vi "main 1.12 stable LR.vi"() -> ()   [LabVIEW 2020]
uses:
  subvi/Newport ESP301/Newport ESP301.lvlib
  subvi/sp_manip.llb/sp_manip_lib.lvlib
  subvi/sp_manip.llb/tcp_gateway.lvlib
  subvi/PHOIBOS/DEFINITIONS/DEF_dev_type.ctl
  subvi/PHOIBOS/DEFINITIONS/DEF_dev_state.ctl
  <vilib>/Utility/file.llb/Write Delimited Spreadsheet (DBL).vi
  <vilib>/Analysis/NI_AALBase.lvlib
  <vilib>/Analysis/1siggen.llb/Ramp Pattern by Samples.vi
  <vilib>/Analysis/NI_AALPro.lvlib
  <vilib>/Analysis/_algsub.llb/Real Vector Norm.vi
  subvi/ZaberTSeries/ZaberTSeries.lvlib
  <vilib>/Utility/file.llb/Write Delimited Spreadsheet (string).vi
  <vilib>/DAQmx/create/channels.llb/DAQmx Create Channel (DI-Digital Input).vi
  <vilib>/Utility/file.llb/Read Delimited Spreadsheet (string).vi
panel:
  out "Pics L":i32=20
  out "Waveform Chart":dbl(graph)
  out "G2 X":cluster{dbl[], "Ramp Pattern":dbl[]}(graph)
  in  "reset every n pics":bool=TRUE
  in  "pics2avg":i32=50
  in  "abort acq.":bool
  out "G2 Y":cluster{dbl[], "Ramp Pattern":dbl[]}(graph)
  out "ETA":timestamp=timestamp(3553173084.423481 s since 1904-01-01) format="%<%H:%M:%S>T"
  out "acq. imgs":i32=20
  out "snap_prog":dbl(slide)=1.0 scale=0.0..1.0
  in  "BasePath":path=path "Z:/PESdata"
  in  "cam_liveavg":bool=TRUE caption="live average"
  out "cam_fps":dbl=19.778711584654577 caption="FPS" format="%.1g"
  out "sideimg":dbl[][](graph)
  out "RunNumber":u16=1876
  out "sum":dbl format="%#.2g"
  out "max":dbl
  out "mainimg":dbl[][](graph)
  out "ESP_con?":bool=TRUE caption="ESP301"
  out "phoib_con?":bool caption="PHOIBOS"
  out "manip_con?":bool=TRUE caption="manipulator"
  out "cam_con?":bool caption="camera"
  in  "main_close":bool
  in  "Tab Control":enum32{"live", "1D scan", "devices"}(tab)=enum."devices"
  in  "phoib_I_10s":dbl=0.0039
  out "phoib_I_10":dbl caption="Mesh Back"
  in  "mirr_go":bool
  in  "ESP_opent0file":bool
  in  "mirr_rel":i32=20 caption="relative [steps]"
  in  "mirr_Y-":bool
  in  "mirr_Y+":bool
  in  "mirr_X+":bool
  in  "mirr_X-":bool
  in  "manip_deltas":dbl[](array[numeric])=[0.0, 0.0, 5.0, 0.0, 0.0, 0.0] caption="delta" format="%#.5g"
  in  "aq.mode":enum32{"Radio Selection 1", "Radio Selection 2"}(radio)=enum."Radio Selection 2"
  in  "dark avg":i32=100
  in  "cam_avgs":i32=20 caption="N"
  in  "ESP_delta":dbl caption="relative [mm]"
  in  "ESP_-":bool
  in  "ESP_+":bool
  in  "ESP_go":bool
  in  "ESP_dest_t":dbl=-12656.75602819869 caption="[fs]"
  in  "ESP_dest":dbl=25.0 caption="[mm]"
  in  "ESP_set_t0":bool
  in  "phoib_I_6s":dbl=3200.0
  in  "phoib_I_5s":dbl=1500.0
  in  "phoib_I_4s":dbl=4.558
  in  "phoib_I_3s":dbl=-7.0
  in  "phoib_I_2s":dbl=30.0
  in  "phoib_I_1s":dbl=18.0
  in  "phoib_standby":bool
  in  "phoib_set":bool
  out "phoib_I_6":dbl caption="Screen Voltage"
  out "phoib_I_5":dbl caption="Detctor Voltage"
  out "phoib_I_4":dbl caption="Work Function"
  out "phoib_I_3":dbl caption="Coil Current"
  out "phoib_I_2":dbl caption="Pass Energy"
  out "phoib_I_1":dbl caption="Kinetic Energy"
  out "Saved Positions":string[][](table)=[["ertwertwert", "-2.299945", "-2.030214", "38.900024", "50.000762", "0.000887", "-97.998082"], ["uztgugt", "-14.999451", "-13.638894", "442.380066", "13.998380", "-1.893758", "-76.305838"], ["asdf", "-14.999451", "-13.638894", "442.380066", "13.998380", "-1.893758", "-76.305838"], ["test3", "-14.999451", "-13.638894", "441.380066", "13.998380", "-1.893758", "-76.305838"]]
  in  "Save Pos":bool
  in  "Load":bool
  in  "Delete":bool
  in  "ManipRel +":bool
  in  "ManipRel -":bool
  in  "Move Abs":bool
  in  "stop manip":bool
  in  "dest":dbl[](array[numeric])=[-0.09886108403264701, -4.840202394941505, 34.40008544921875, 285.0011913575033, -7.998926328051604, 138.99937717186526] caption="destination" format="%#.5g"
  out "axis":string[](array[string])=["x", "y", "z", "polar", "tilt", "azimut"]
  out "pos":dbl[](array[numeric])=[-0.09886108403264701, -4.840202394941505, 34.40008544921875, 285.0011913575033, -7.998926328051604, 138.99937717186526] caption="position" format="%.5f"
  in  "ana_mode":T1(ring)=enum."WideAngleMode"
  in  "ana_voltrange":enum16{"3.5kV", "1.5kV", "400V", "100V", "10V"}(ring)=enum."400V"
  out "ESP_pos":dbl=nan caption="Position"
  out "ESP_delay":dbl=nan caption="Delay"
  out "ESP_t0":dbl=25.0 caption="Time Zero @"
  out "phoib_I_7":dbl caption="Conversion Voltage"
  in  "phoib_I_7s":dbl=-26.0
  in  "phoib_I_8s":dbl=0.0039
  in  "phoib_I_9s":dbl=0.0039
  out "phoib_I_8":dbl caption="FD1"
  out "phoib_I_9":dbl caption="Mesh Front"
  in  "gain":bool
  in  "cam_exp":u32=50 caption="exposure [ms]"
  in  "binning":u16(ring)=2 items=["X 1", "X 2", "X 4", "X 8"]
  in  "cam_dark?":bool=TRUE caption="subtract dark?"
  in  "cam_dark":bool
  in  "cam_saveimg":bool
  in  "e-size":u8
  in  "lower threshold":i32=50
  in  "count?":bool
  in  "ROI Left":i32=1
  in  "ROI Right":i32=43
  in  "ROI Top":i32=1
  in  "ROI Bottom":i32=33
  out "moving?":bool[](array[boolean])
  out "mirr_posX":i32=-142 caption="X"
  out "mirr_posY":i32=4922 caption="Y"
  in  "mirr_dest":i32[](array[numeric])=[-64, -2601]
  out "anglegraph":dbl[][](graph)
  out "intensitygraph":cluster{"Array":dbl[], "Intensity Chart":dbl[]}(graph)={"Array"=[-100000.0, -95000.0, -90000.0, -85000.0, -80000.0, -75000.0, -70000.0, -65000.0, -60000.0, -55000.0, -50000.0, -45000.0, -40000.0, -35000.0, -30000.0, -25000.0, -20000.0, -15000.0, -10000.0, -5000.0, 0.0, 5000.0, 10000.0, 15000.0, 20000.0, 25000.0, 30000.0, 35000.0, 40000.0, 45000.0, 50000.0], "Intensity Chart"=[710968.0999999978, 661453.8299999974, 660491.1499999983, 654490.9100000008, 607000.039999999, 668861.0999999981, 631366.7699999984, 739689.6549999982, 681310.9099999986, 658872.4599999987, 692812.8950000014, 671304.7250000003, 670701.9799999978, 684100.4049999971, 706126.3150000001, 744782.0600000009, 684440.8499999981, 704157.155, 756957.4599999988, 768506.4449999956, 761428.5800000022, 678039.9949999974, 735774.9649999988, 659533.465000001, 724648.9199999974, 705546.0750000002, 773026.2399999972, 698578.0149999986, 697856.3899999985, 787613.0450000013, 750231.4800000007]}
  in  "scan_selector":enum32{"delay", "manip", "mirror", "volt"}(tab)
  in  "scan_manip_setstart":bool
  in  "scan_manip_start":dbl[](array[numeric])=[-2.6172862113166087, -0.009888298846365134, 68.5008544921875, -46.363686276590336, 11.108982061941884, -218.56360350415366] caption="start position" format="%#.5g"
  in  "scan_manip_deltas":dbl[](array[numeric])=[0.0, 0.0, 0.0, 0.0, 10.0, 0.0] caption="direction vector\n(gets normed)" format="%#.5g"
  in  "scan_mirr_start":i32[](array[numeric])=[-64, -2601]
  in  "scan_mirr_deltas":i32[](array[numeric])=[0, 0, 0, 0, 10, 0] caption="direction vector\n(gets normed)"
  in  "scan_mirr_setstart":bool
  in  "scan_volt_parameter":string(combo)="Kinetic Energy"
  in  "meas_iter":i32=60 caption="Iterations"
  out "duration [HH:MM:SS]":dbl=4512.494100093842 format="%<%H:%M:%S>t"
  out "disk [MB]":dbl=1028.5800000000002
  out "RAM [MB]":dbl=17.143
  out "total steps":i32=1860
  out "measpoints":i32=31
  in  "load delay table":bool
  in  "scan_go":bool
  in  "waypoints":string[][](table)=[["-100000", "5000"], ["50000", ""], ["", ""]]
  in  "stop after step":bool
  out "scan":dbl(slide)=0.967741935483871 scale=0.0..1.0
  out "iteration":dbl(slide)=0.03333333333333333 scale=0.0..1.0
  out "current scan":i32=30
  out "current iteration":i32=2
  in  "time/step [s]":dbl=2.426072096824646
  in  "stop after iteration":bool
  out "energygraph":dbl[][](graph)
  in  "mirr_init":bool
  in  "mirr_release":bool
  in  "mirr_Y#":u8=2
  in  "manip_init":bool
  in  "manip_release":bool
  in  "phoib_init":bool
  in  "phoib_release":bool
  in  "ESP_init":bool
  in  "ESP_release":bool
  in  "ESP301 VISA":refnum<visa-resource-name>="COM9"
  in  "board number":i32
  in  "cam_init":bool
  in  "cam_release":bool
  out "cam_error":errorcluster
  out "phoib_error":errorcluster
  out "state":T2 items=["Off"=-1, "Standby"=0, "On"=1]
  in  "ESP Axis":i32=3 min=1 max=3
  out "error out":errorcluster={"status"=FALSE, "code"=1073676418, "source"="VISA Close in Newport ESP301.lvlib:Close.vi->main 1.12 stable LR.vi"}
  out "error out 2":errorcluster={"status"=TRUE, "code"=1, "source"="TCP Write in sp_manip_lib.lvlib:sp_manip_disconnect.vi->main 1.12 stable LR.vi"}
  out "mirr_Error":errorcluster={"status"=FALSE, "code"=1073676418, "source"="VISA Close in ZaberTSeries.lvlib:Close.vi->main 1.12 stable LR.vi"}
  in  "mirr_VISA":refnum<visa-resource-name>="COM7"
  in  "mirr_X#":u8=1
  in  "Operating mode\nHP & QE / HS & DiCam Pro":u32=1
  in  "Frame trigger \n(High Performance and QE only)":u16
  # "camera"
  # "analyzer"
  # "manipulator"
  # "aquisition"
  # "delay stage"
  # "mirror"
  # "Position"
  # "Destination"
  # "- no settings -"
  # "waypoints are absolute values"
  # "X\nY\nZ\npolar\ntilt\nazimut"
  # "waypoint \"0\" is start position"
  # "X\nY"
  # "waypoint \"0\" is start position"
  # "waypoints are absolute values"
  # "camera"
  # "phoibos"
  # "ESP301"
  # "manipulator"
  # "mirror"
  # "0 = sequential\n1 = simultaneous"
  # "0 = internal\n1 = external rising\n2 = external falling"
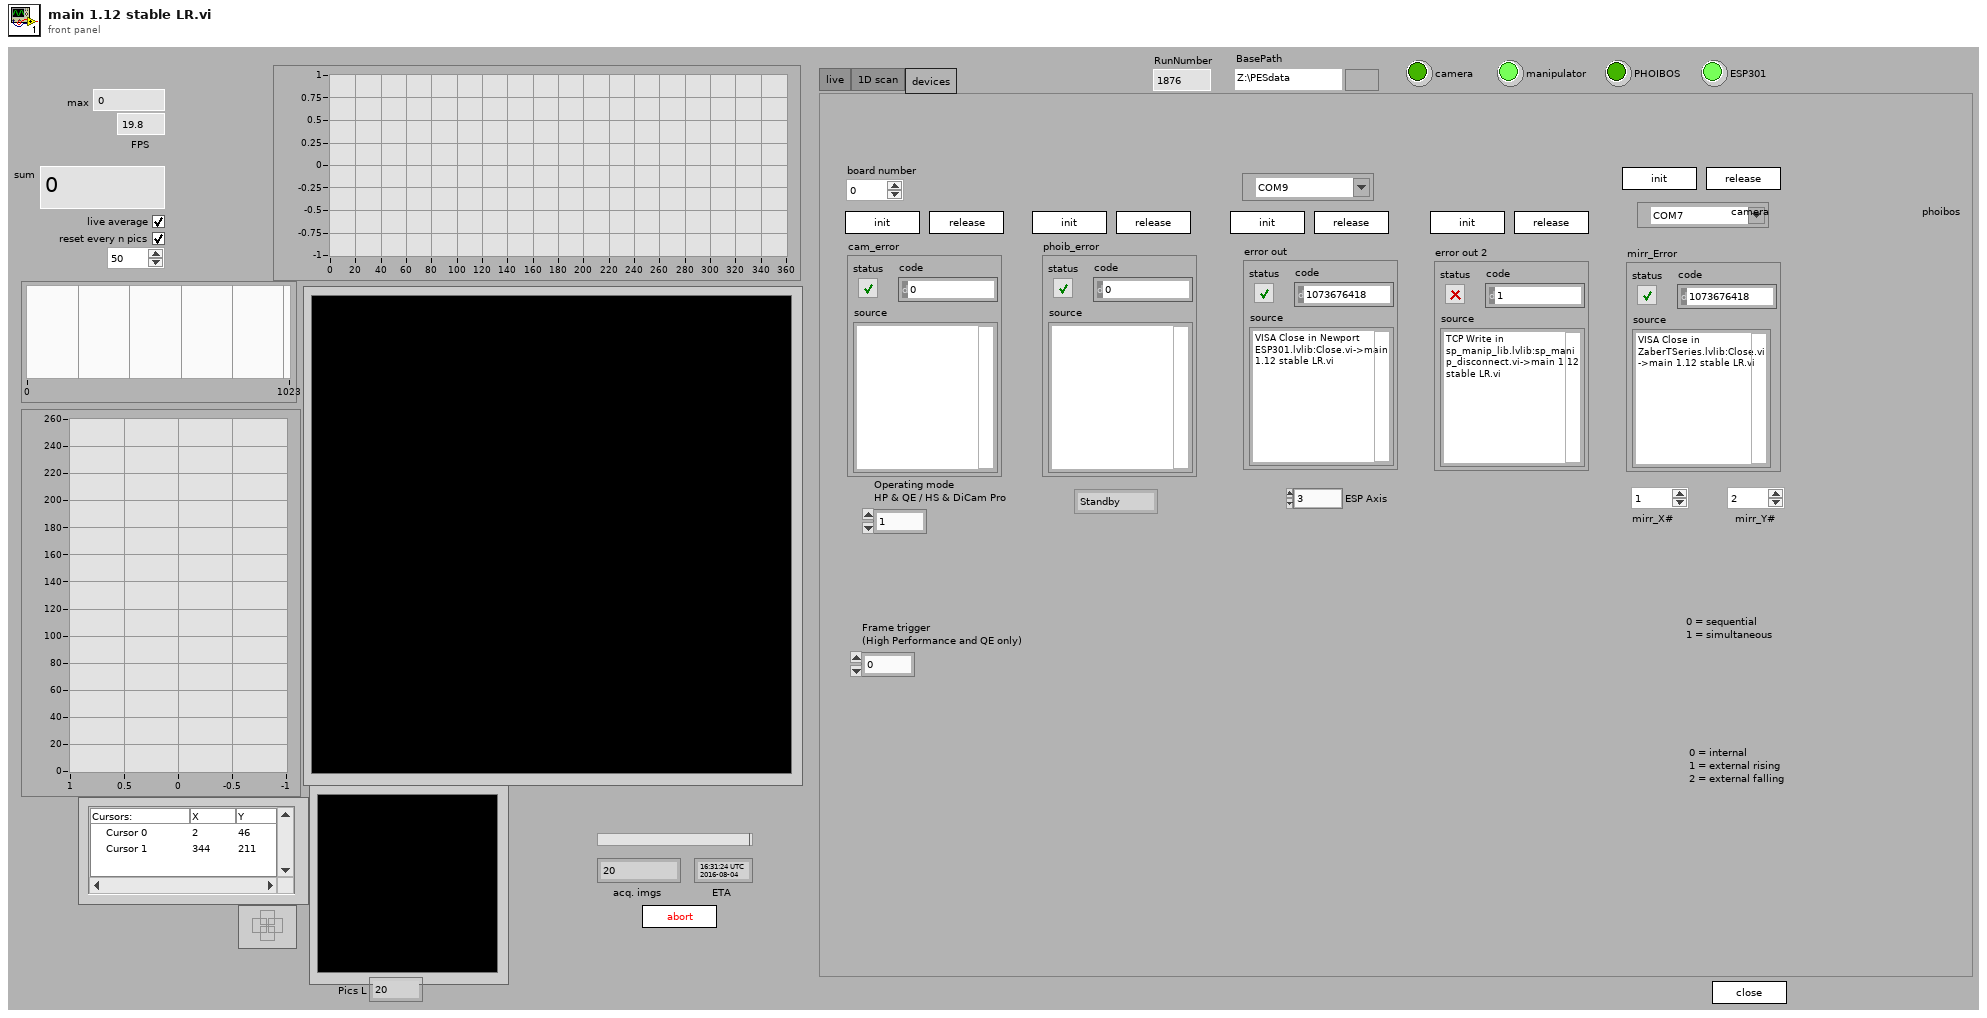
[diagram p1: front panel]
types:
  T1 = enum16{"HighMagnification", "MediumMagnification", "LowMagnification", "HighAngularDispersion", "MediumAngularDispersion", "LowAngularDispersion", "WideAngleMode", "LargeArea", "MediumArea", "SmallArea", "HighMagnification2", "SmallArea2"}
  T2 = typedef "DEF_dev_state.ctl" = i32
  T3 = cluster{"queue out":refnum<queue>, "queue out":refnum<queue>, "queue out":refnum<queue>, "queue out":refnum<queue>, "queue out":refnum<queue>}
  T4 = typedef "LVCursorListTypeDef.ctl" = cluster{"Name":string, "Color":u32, "Style":u8, "Point Style":u8, "Name Visible":bool, "Allow Drag":bool, "Cursor Mode":u32, "Plot":i32, "Index":i32, "Position":cluster{"X":dbl, "Y":dbl}, "X Scale":u32, "Y Scale":u32, "Watch Plots":i32[], "Watch All Plots":bool, "Plot Area":i32, "Label Offset":cluster{"X":dbl, "Y":dbl}}[]
  T5 = cluster{"Camera type":u32, "Operating mode\nHP & QE / HS & DiCam Pro ":u32, "Frame trigger \n(High Performance and QE only)":u16, "Sequence trigger":u16, "Low Light\n(QE only)":bool, "Gain":bool, "Horzontal\nbinning":u16, "Vertical\nbinning ":u16, "ROI Left":i32, "ROI Right":i32, "ROI Top":i32, "ROI Bottom":i32}
  T6 = cluster{"Name":string, "Color":u32, "Style":u8, "Point Style":u8, "Name Visible":bool, "Allow Drag":bool, "Cursor Mode":u32, "Plot":i32, "Index":i32, "Position":cluster{"X":dbl, "Y":dbl}, "X Scale":u32, "Y Scale":u32, "Watch Plots":i32[], "Watch All Plots":bool, "Plot Area":i32, "Label Offset":cluster{"X":dbl, "Y":dbl}}
  T7 = cluster{"mirr_X#":u8, "Command":u8, dbl, "Response Count":i32}
  T8 = cluster{"mirr_Y#":u8, "Command":u8, dbl, "Response Count":i32}
  T9 = cluster{i32, "Command":u8, i32, "Response Count":i32}
  T10 = cluster{"Axis_Name":string, "Axis_Type":string, "Axis_Position":dbl, "continous":bool, "moving":bool}[]
  T11 = typedef "DEF_dev_type.ctl" = enum32{"devA (analyzer)", "devD (detector)"}
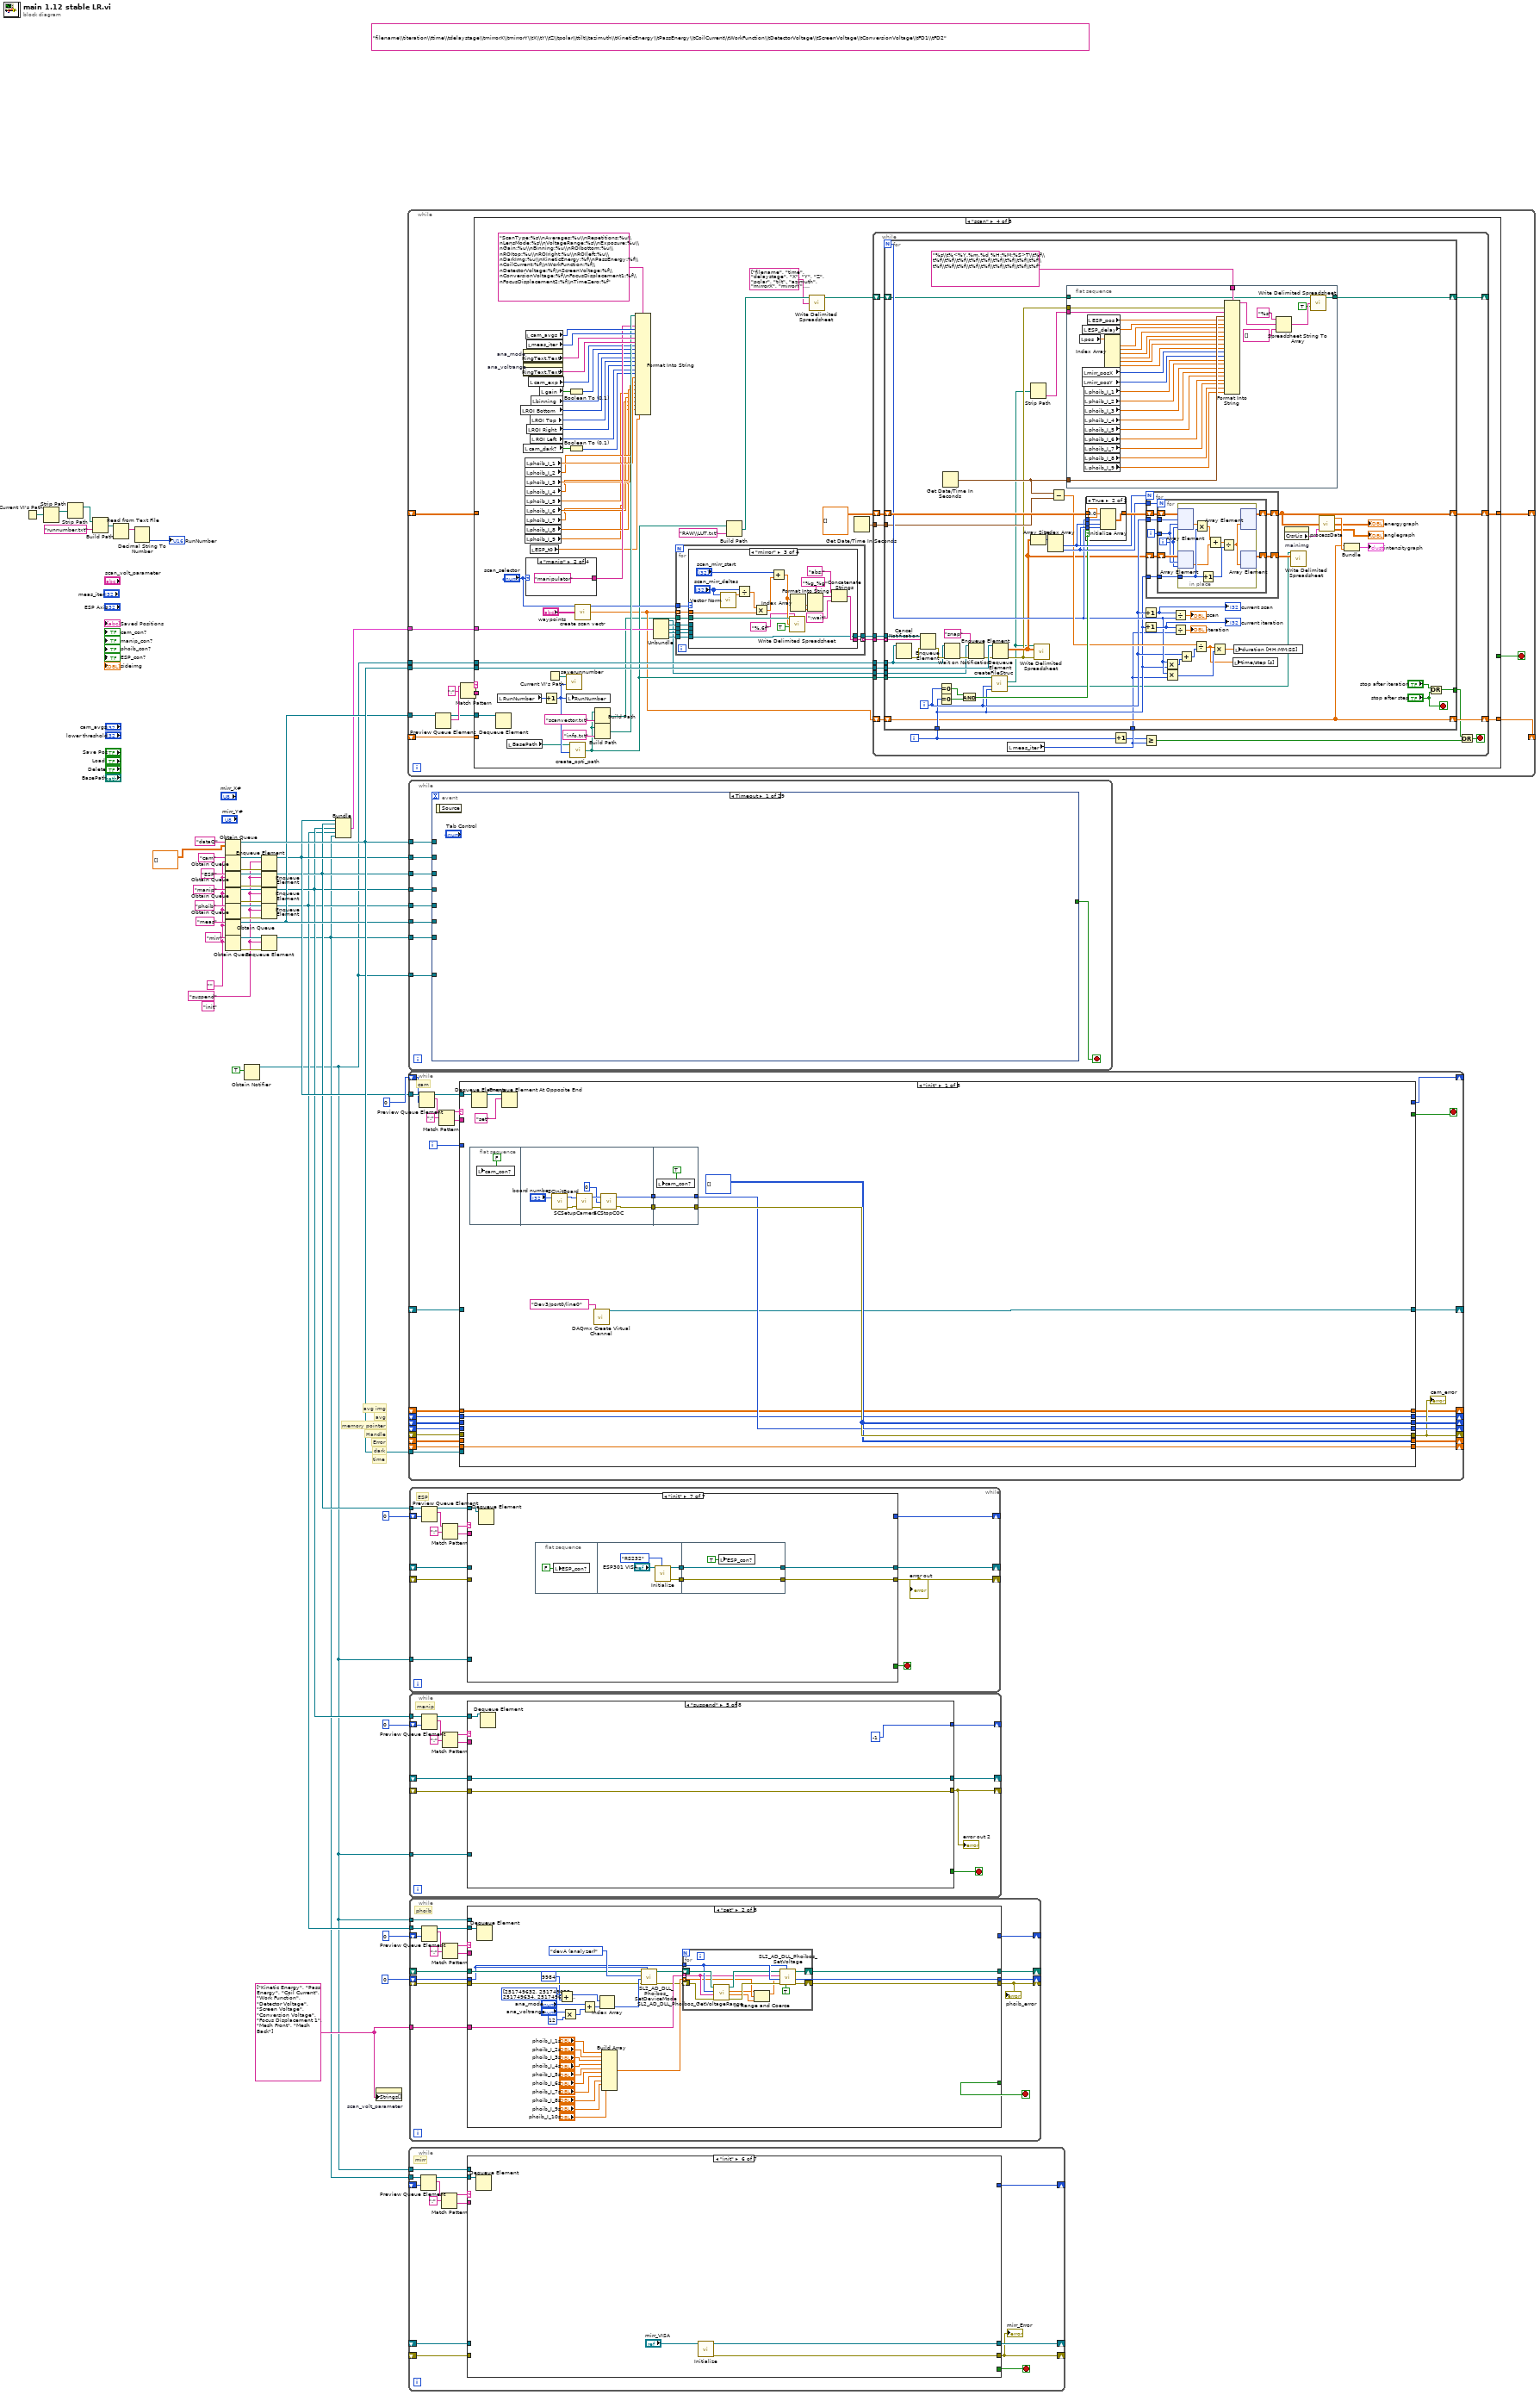
[diagram p0: block diagram]
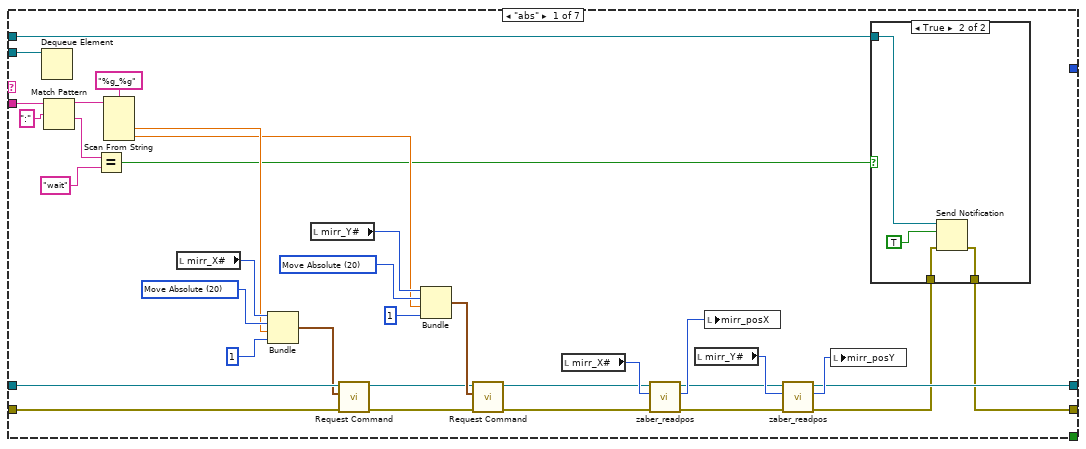
[diagram p2: hidden frame]
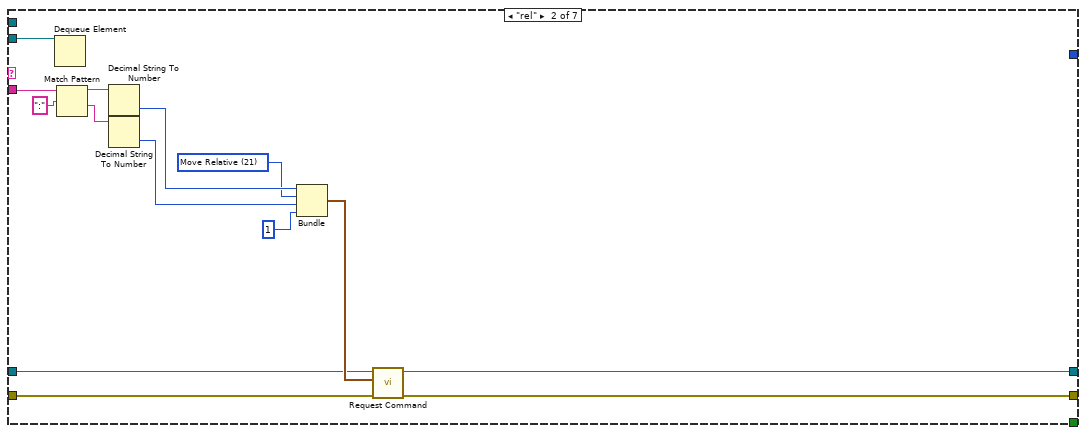
[diagram p4: hidden frame]
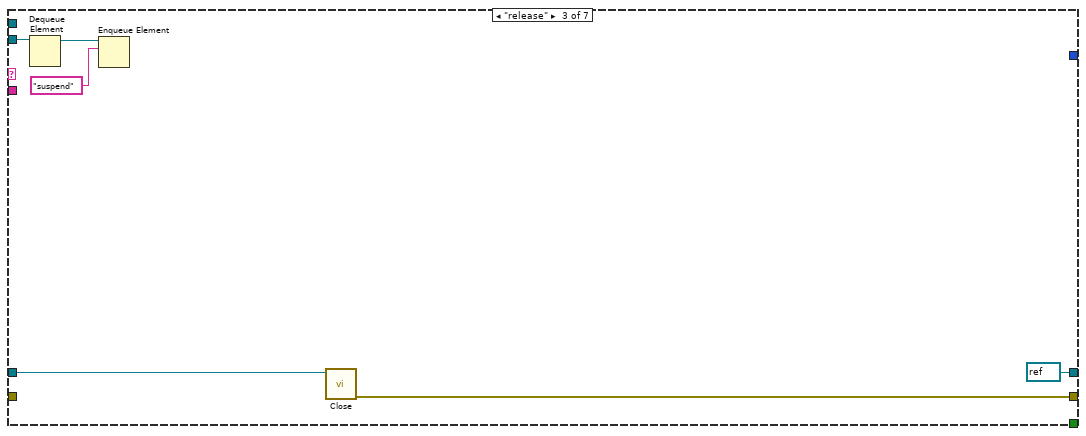
[diagram p5: hidden frame]
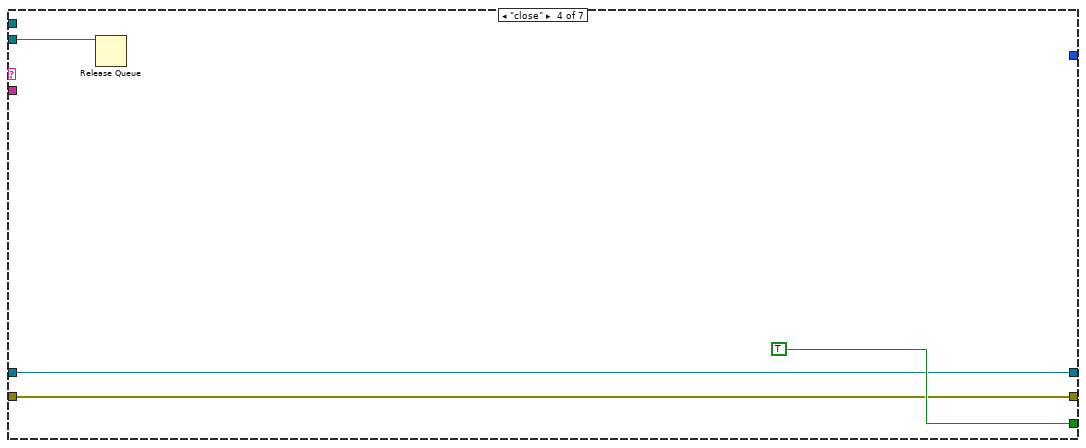
[diagram p6: hidden frame]
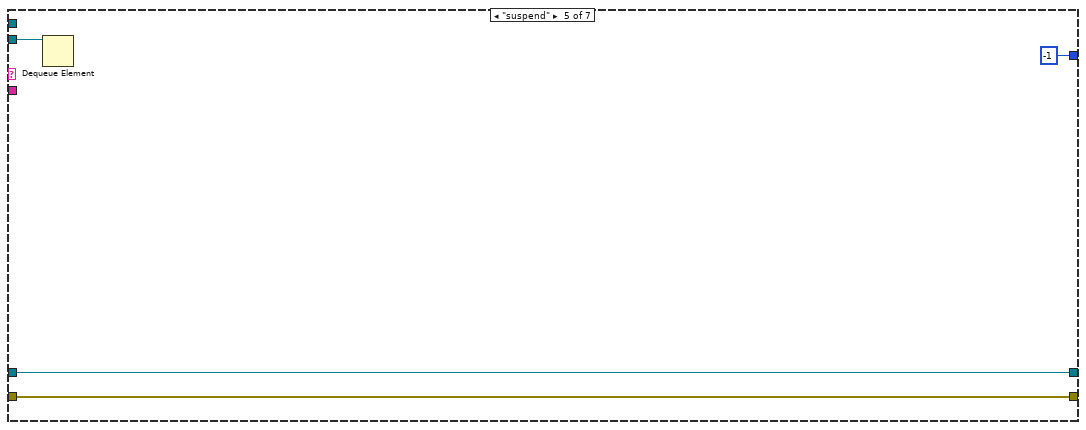
[diagram p7: hidden frame]
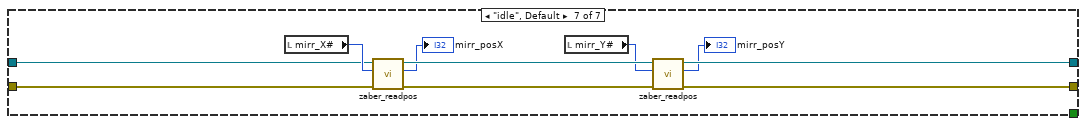
[diagram p8: hidden frame]
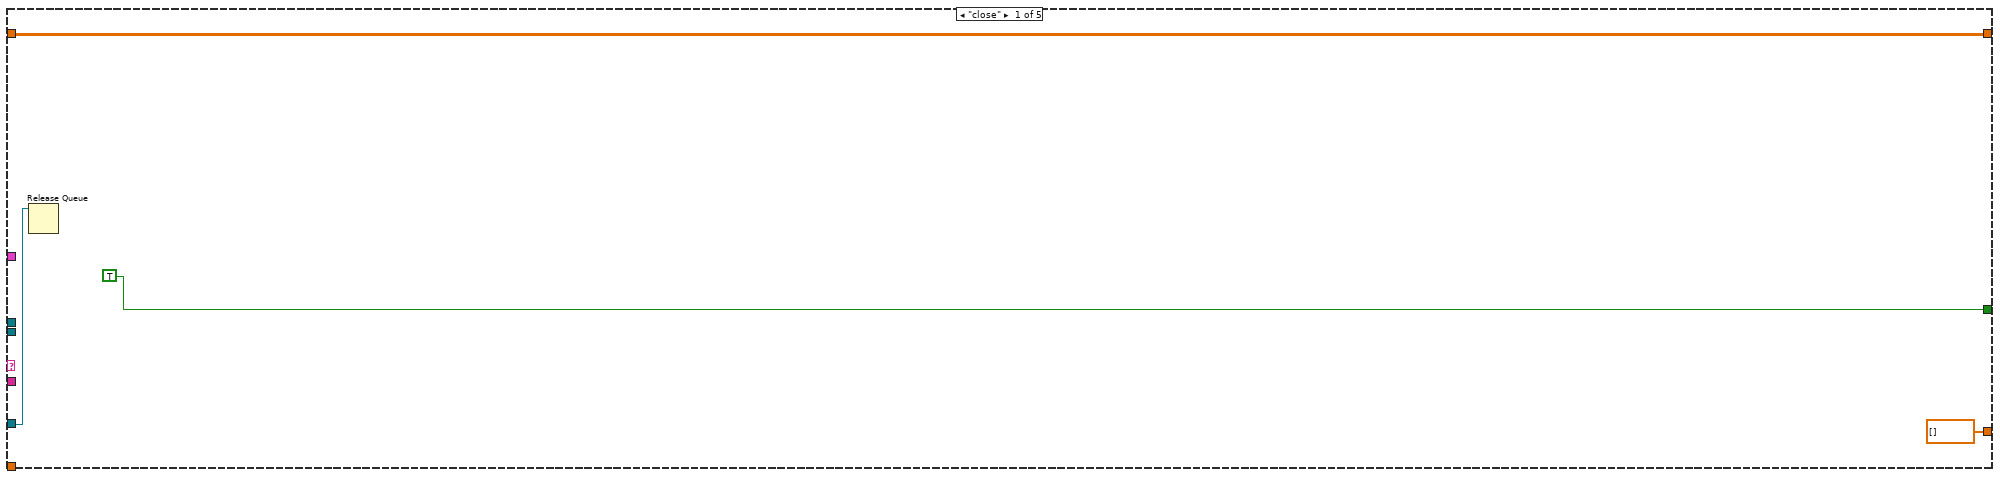
[diagram p9: hidden frame]
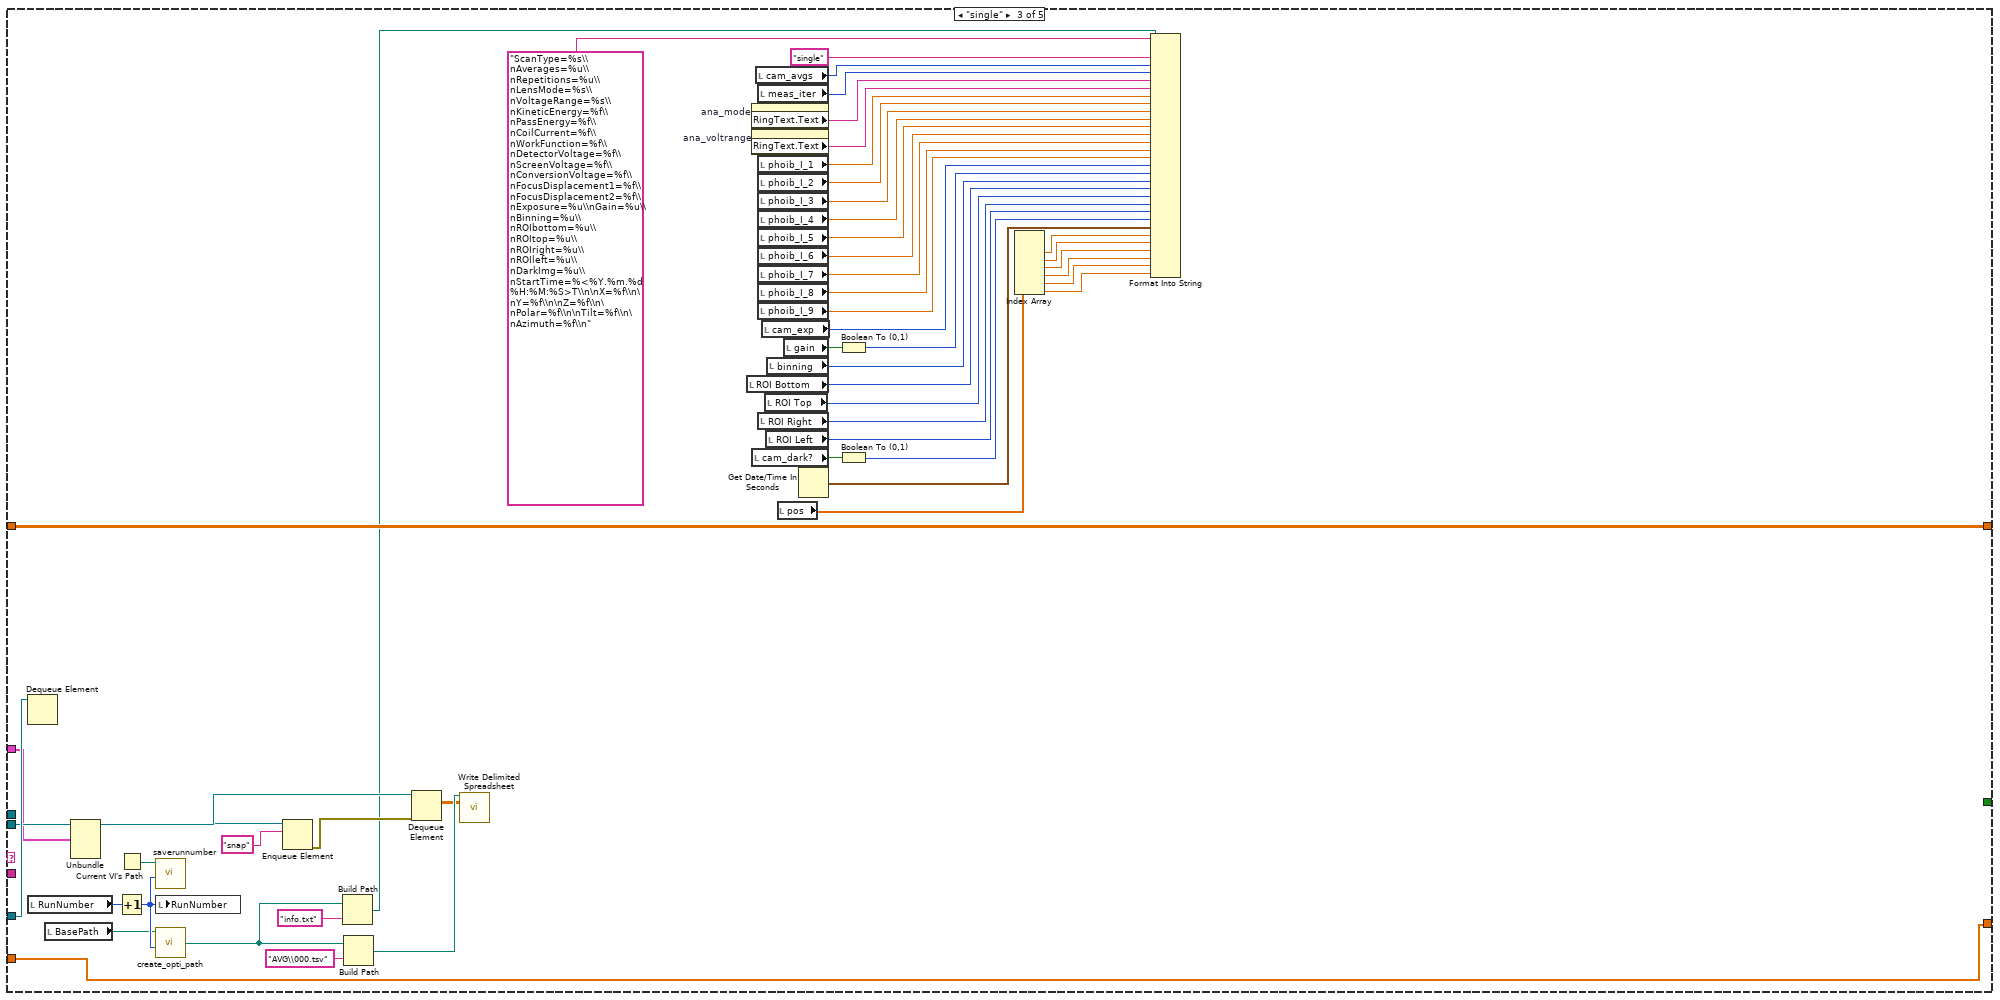
[diagram p11: hidden frame]
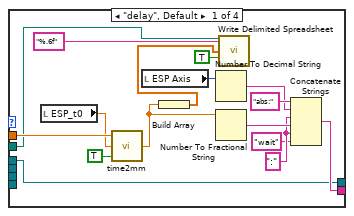
[diagram p13: hidden frame]
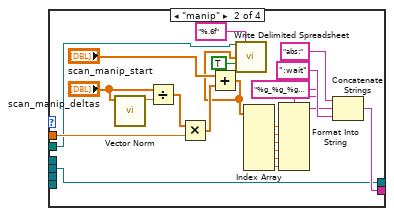
[diagram p14: hidden frame]
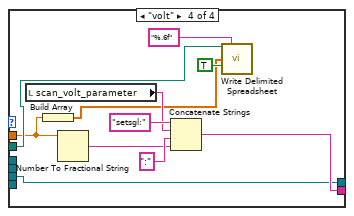
[diagram p15: hidden frame]
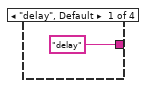
[diagram p16: hidden frame]
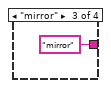
[diagram p17: hidden frame]
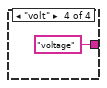
[diagram p18: hidden frame]
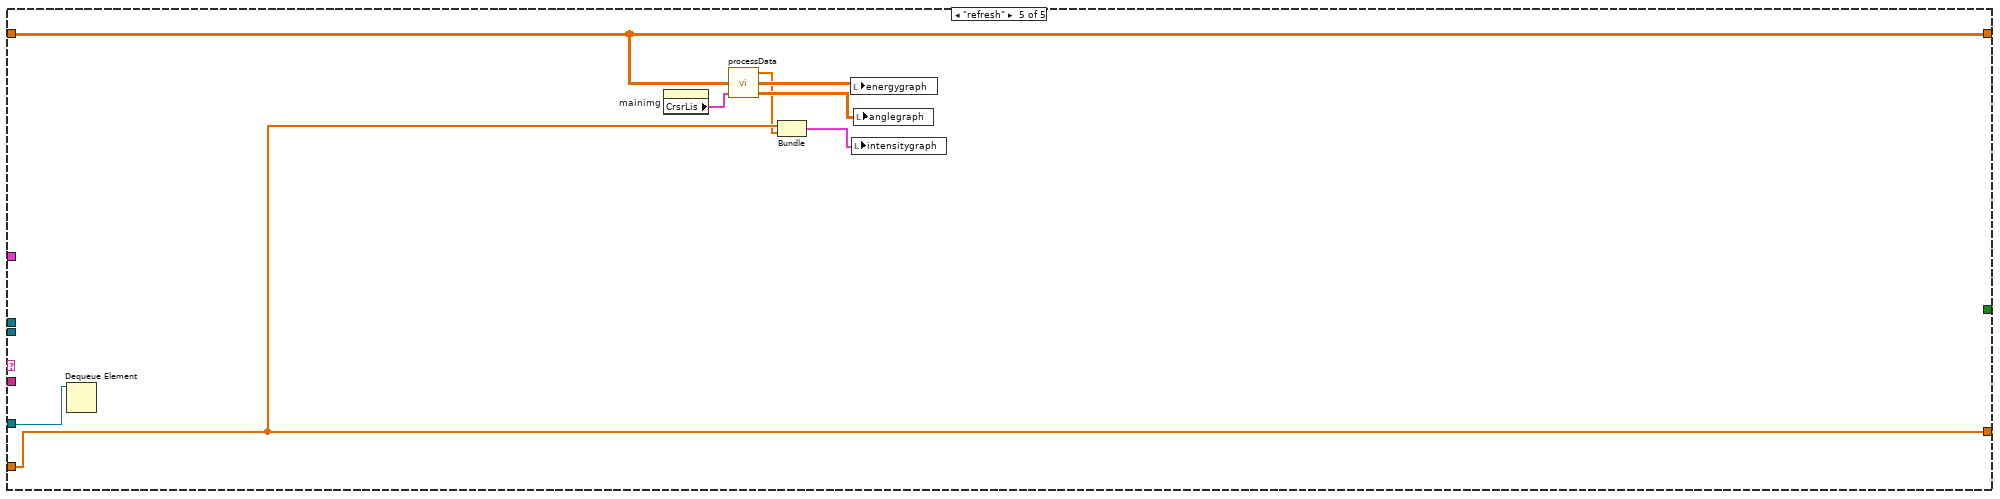
[diagram p19: hidden frame]
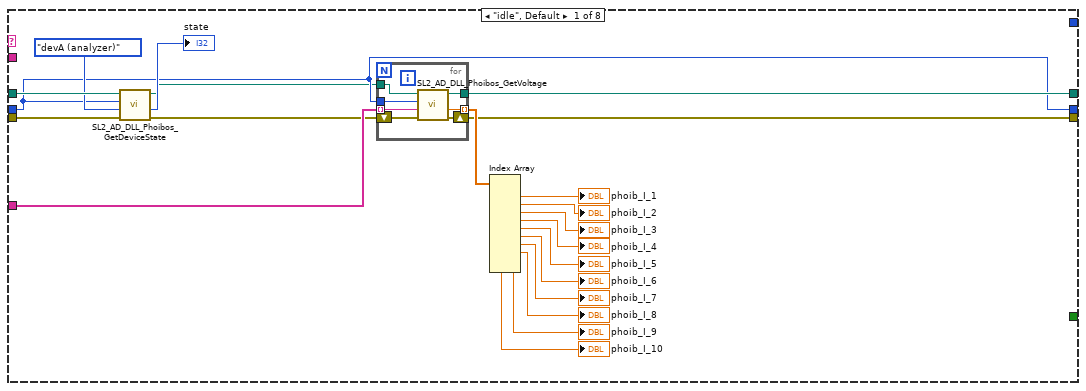
[diagram p20: hidden frame]
diagram:
  (unwired) "filename\\titeration\\ttime\\tdelaystage\\tmirrorX\\tmirrorY\\tX\\tY\\tZ\\tpolar\\ttilt\\tazimuth\\tKineticEnergy\\tPassEnergy\\tCoilCurrent\\tWorkFunction\\tDetectorVoltage\\tScreenVoltage\\tConversionVoltage\\tFD1\\tFD2"
  w9 = string[] ["Kinetic Energy", "Pass Energy", "Coil Current", "Work Function", "Detector Voltage", "Screen Voltage", "Conversion Voltage", "Focus Displacement 1", "Mesh Front", "Mesh Back"]
  (unwired) "init" ("name (unnamed)")
  w1 = "suspend" ("name (unnamed)")
  w2 = "" ("name (unnamed)")
  # "avg img"
  # "avg"
  # "time"
  # "dark"
  # "Error"
  # "Handle"
  # "memory pointer"
  n1 = Current VI's Path() -> (path=w17:path)
  n2 = Strip Path(path=w17) -> (stripped path=w21:path)  [unwired: 1 out]
  n3 = Strip Path(path=w21) -> (stripped path=w22:path)  [unwired: 1 out]
  n4 = Build Path(base path=w22, name or relative path="runnumber.txt") -> (appended path=w19:path)
  n5 = Read from Text File(file (use dialog)=w19) -> (text=w20:string)  [unwired: 3 in, 3 out]
  n6 = Decimal String To Number(string=w20) -> (number=→"RunNumber":i32)  [unwired: 2 in, 1 out]
  n7 = Obtain Queue(name (unnamed)="dataQ", element data type=dbl[][] []) -> (queue out=w23:refnum<queue>)  [unwired: 3 in, 2 out]
  n8 = Obtain Queue(name (unnamed)="cam", element data type=w2) -> (queue out=w42:refnum<queue>, error out=w41:errorcluster)  [unwired: 3 in, 1 out]
  n9 = Obtain Queue(name (unnamed)="ESP", element data type=w2) -> (queue out=w39:refnum<queue>, error out=w40:errorcluster)  [unwired: 3 in, 1 out]
  n10 = Obtain Queue(name (unnamed)="manip", element data type=w2) -> (queue out=w36:refnum<queue>, error out=w35:errorcluster)  [unwired: 3 in, 1 out]
  n11 = Obtain Queue(name (unnamed)="phoib", element data type=w2) -> (queue out=w33:refnum<queue>, error out=w34:errorcluster)  [unwired: 3 in, 1 out]
  n12 = Obtain Queue(name (unnamed)="meas", element data type=w2) -> (queue out=w16:refnum<queue>)  [unwired: 3 in, 2 out]
  n13 = Obtain Queue(name (unnamed)="mirr", element data type=w2) -> (queue out=w7:refnum<queue>, error out=w6:errorcluster)  [unwired: 3 in, 1 out]
  n14 = Obtain Notifier(notification data type=TRUE) -> (notifier out=w3:refnum<notifier>)  [unwired: 3 in, 2 out]
  n15 = Enqueue Element(queue=w42, element=w1, error in (no error)=w41) -> (queue out=w14:refnum<queue>)  [unwired: 1 in, 2 out]
  n16 = Enqueue Element(queue=w39, element=w1, error in (no error)=w40) -> (queue out=w13:refnum<queue>)  [unwired: 1 in, 2 out]
  n17 = Enqueue Element(queue=w36, element=w1, error in (no error)=w35) -> (queue out=w12:refnum<queue>)  [unwired: 1 in, 2 out]
  n18 = Enqueue Element(queue=w33, element=w1, error in (no error)=w34) -> (queue out=w11:refnum<queue>)  [unwired: 1 in, 2 out]
  n19 = Enqueue Element(queue=w7, element=w1, error in (no error)=w6) -> (queue out=w4:refnum<queue>)  [unwired: 1 in, 2 out]
  n20 = Bundle("queue out"=w14, "queue out"=w13, "queue out"=w12, "queue out"=w11, "queue out"=w4) -> (w15:T3)  [unwired: 1 in]
  n21 = property on="scan_volt_parameter" class="CmbBox"("Strings[]"=w9) -> ()  [unwired: 2 in, 2 out]
  n22 = while {
    tunnel: w23 -> [w57]
    tunnel: w16 -> [w54]
    tunnel: w15 -> [w50]
    shift-right: [w48] -> _
    shift-left: _ -> [w47]
    tunnel: w3 -> [w46]
    shift-right: [w45] -> _
    shift-left: _ -> [w44]
    stop <- w49 stop-if-true
    n23 = Preview Queue Element(queue=w54) -> (queue out=w51:refnum<queue>, element=w56:string)  [unwired: 2 in, 2 out]
    n24 = Match Pattern(string=w56, regular expression=":") -> (before substring=w53:string, after substring=w52:string)  [unwired: 1 in, 2 out]
    n25 = case shown="\"scan\"" w53 {
      tunnel: w57 -> [_ _ w113 w165 _]
      tunnel: w52 -> [_ _ _ _ _]
      tunnel: w51 -> [w61 _ w114 w161 w385]
      tunnel: [TRUE _ _ _ _] -> w49
      tunnel: w50 -> [_ _ w101 w141 _]
      tunnel: [w59 w63 w99 w163 w391] -> w48
      tunnel: w47 -> [w59 w63 w99 _ w391]
      tunnel: w46 -> [_ _ _ w162 _]
      tunnel: [dbl[] [] ("Array") w62 w71 w127 w387] -> w45
      tunnel: w44 -> [_ w62 w71 _ w387]
      frame "close" {
        n26 = Release Queue(queue=w61) -> ()  [unwired: 2 in, 3 out]
      }
      frame "idle", Default {
      }
      frame "single" {
        n27 = Dequeue Element(queue=w114) -> ()  [unwired: 2 in, 4 out]
        n28 = local read "RunNumber"() -> (w108:u16)
        n29 = local read "BasePath"() -> (w109:path)
        n30 = Unbundle(w101) -> ("queue out"=w100:refnum<queue>)  [unwired: 4 out]
        n31 = Increment(x=w108) -> (x+1=w110:u16)
        n32 = Current VI's Path() -> (path=w107:path)
        n33 = call "saverunnumber.vi"("RunNumber"=w110, "VI path"=w107) -> ()  [unwired: 10 in]
        n34 = local write "RunNumber"(w110) -> ()
        n35 = call "create_opti_path.vi"("RunNumber"=w110, "base path"=w109) -> ("Path"=w103:path)  [unwired: 2 in]
        n36 = Enqueue Element(queue=w100, element="snap" ("string")) -> (error out=w111:errorcluster)  [unwired: 2 in, 2 out]
        n37 = Build Path(base path=w103, name or relative path="info.txt") -> (appended path=w72:path)
        n38 = Build Path(base path=w103, name or relative path="AVG\\000.tsv") -> (appended path=w105:path)
        n39 = Dequeue Element(queue=w113, error in (no error)=w111) -> (element=w102:dbl[][])  [unwired: 1 in, 3 out]
        n40 = call-poly <vilib>:"Write Delimited Spreadsheet.vi"("file path (dialog if empty)"=w105, "2D data"=w102) -> ()  [unwired: 12 in, 2 out]
        n41 = local read "ROI Bottom"() -> (w79:i32)
        n42 = property on="ana_mode" class="Enum (strict)"() -> ("RingText.Text"=w94:string)  [unwired: 2 in, 2 out]
        n43 = property on="ana_voltrange" class="Enum (strict)"() -> ("RingText.Text"=w93:string)  [unwired: 2 in, 2 out]
        n44 = local read "cam_dark?"() -> (w75:bool)
        n45 = local read "cam_avgs"() -> (w96:i32)
        n46 = local read "meas_iter"() -> (w95:i32)
        n47 = local read "phoib_I_1"() -> (w92:dbl)
        n48 = local read "phoib_I_2"() -> (w91:dbl)
        n49 = local read "phoib_I_3"() -> (w90:dbl)
        n50 = local read "phoib_I_4"() -> (w89:dbl)
        n51 = local read "phoib_I_5"() -> (w88:dbl)
        n52 = local read "phoib_I_6"() -> (w87:dbl)
        n53 = local read "phoib_I_7"() -> (w86:dbl)
        n54 = local read "phoib_I_8"() -> (w85:dbl)
        n55 = local read "phoib_I_9"() -> (w84:dbl)
        n56 = local read "ROI Right"() -> (w77:i32)
        n57 = local read "cam_exp"() -> (w83:u32)
        n58 = local read "ROI Top"() -> (w78:i32)
        n59 = local read "ROI Left"() -> (w76:i32)
        n60 = local read "binning"() -> (w80:u16)
        n61 = local read "pos"() -> (w70:dbl[])
        n62 = local read "gain"() -> (w82:bool)
        n63 = Get Date/Time In Seconds() -> (seconds since 1Jan1904=w73:timestamp)
        n64 = Boolean To (0,1)(Boolean=w82) -> (0, 1=w81:i16)
        n65 = Boolean To (0,1)(Boolean=w75) -> (0, 1=w74:i16)
        n66 = Index Array(array=w70) -> (element #1=w69:dbl, element #2=w68:dbl, element #3=w67:dbl, element #4=w66:dbl, element #5=w65:dbl, element #6=w64:dbl)  [unwired: 6 in]
        n67 = Format Into String(format string="ScanType=%s\\nAverages=%u\\nRepetitions=%u\\nLensMode=%s\\nVoltageRange=%s\\nKineticEnergy=%f\\nPassEnergy=%f\\nCoilCurrent=%f\\nWorkFunction=%f\\nDetectorVoltage=%f\\nScreenVoltage=%f\\nConversionVoltage=%f\\nFocusDisplacement1=%f\\nFocusDisplacement2=%f\\nExposure=%u\\nGain=%u\\nBinning=%u\\nROIbottom=%u\\nROItop=%u\\nROIright=%u\\nROIleft=%u\\nDarkImg=%u\\nStartTime=%<%Y.%m.%d %H:%M:%S>T\\n\nX=%f\\n\nY=%f\\n\nZ=%f\\n\nPolar=%f\\n\nTilt=%f\\n\nAzimuth=%f\\n", initial string=w72, "single" ("input 1"), w96, w95, w94, w93, w92, w91, w90, w89, w88, w87, w86, w85, w84, w83, w81, w80, w79, w78, w77, w76, w74, w73, w69, w68, w67, w66, w65, w64) -> ()  [unwired: 1 in, 2 out]
      }
      frame "scan" {
        n68 = Dequeue Element(queue=w161) -> ()  [unwired: 2 in, 4 out]
        n69 = local read "RunNumber"() -> (w169:u16)
        n70 = local read "BasePath"() -> (w170:path)
        n71 = local read "ROI Bottom"() -> (w147:i32)
        n72 = property on="ana_mode" class="Enum (strict)"() -> ("RingText.Text"=w156:string)  [unwired: 2 in, 2 out]
        n73 = property on="ana_voltrange" class="Enum (strict)"() -> ("RingText.Text"=w155:string)  [unwired: 2 in, 2 out]
        n74 = local read "cam_dark?"() -> (w153:bool)
        n75 = local read "phoib_I_1"() -> (w125:dbl)
        n76 = local read "phoib_I_2"() -> (w124:dbl)
        n77 = local read "phoib_I_3"() -> (w123:dbl)
        n78 = local read "phoib_I_4"() -> (w122:dbl)
        n79 = local read "phoib_I_5"() -> (w121:dbl)
        n80 = local read "phoib_I_6"() -> (w120:dbl)
        n81 = local read "phoib_I_7"() -> (w119:dbl)
        n82 = local read "phoib_I_8"() -> (w118:dbl)
        n83 = local read "phoib_I_9"() -> (w117:dbl)
        n84 = local read "cam_avgs"() -> (w158:i32)
        n85 = case shown="\"manip\"" "scan_selector" {
          tunnel: ["delay" ("input 1") "manipulator" ("input 1") "mirror" ("input 1") "voltage" ("input 1")] -> w151
          frame "delay", Default {
          }
          frame "manip" {
          }
          frame "mirror" {
          }
          frame "volt" {
          }
        }
        n86 = local read "meas_iter"() -> (w157:i32)
        n87 = local read "ROI Right"() -> (w145:i32)
        n88 = local read "cam_exp"() -> (w150:u32)
        n89 = local read "ROI Top"() -> (w146:i32)
        n90 = local read "ESP_t0"() -> (w116:dbl)
        n91 = local read "ROI Left"() -> (w144:i32)
        n92 = local read "binning"() -> (w148:u16)
        n93 = local read "gain"() -> (w154:bool)
        n94 = Increment(x=w169) -> (x+1=w171:u16)
        n95 = Current VI's Path() -> (path=w168:path)
        n96 = call "saverunnumber.vi"("RunNumber"=w171, "VI path"=w168) -> ()  [unwired: 10 in]
        n97 = local write "RunNumber"(w171) -> ()
        n98 = Boolean To (0,1)(Boolean=w154) -> (0, 1=w149:i16)
        n99 = Boolean To (0,1)(Boolean=w153) -> (0, 1=w143:i16)
        n100 = call "create_opti_path.vi"("RunNumber"=w171, "base path"=w170) -> ("Path"=w132:path)  [unwired: 2 in]
        n101 = call "create scan vectr.vi"("Table Control"="waypoints") -> ("Array"=w126:dbl[])
        n102 = Build Path(base path=w132, name or relative path="scanvector.txt") -> (appended path=w115:path)
        n103 = Build Path(base path=w132, name or relative path="info.txt") -> (appended path=w152:path)
        n104 = Format Into String(format string="ScanType:%s\\nAverages:%u\\nRepetitions:%u\\nLensMode:%s\\nVoltageRange:%s\\nExposure:%u\\nGain:%u\\nBinning:%u\\nROIbottom:%u\\nROItop:%u\\nROIright:%u\\nROIleft:%u\\nDarkImg:%u\\nKineticEnergy:%f\\nPassEnergy:%f\\nCoilCurrent:%f\\nWorkFunction:%f\\nDetectorVoltage:%f\\nScreenVoltage:%f\\nConversionVoltage:%f\\nFocusDisplacement1:%f\\nFocusDisplacement2:%f\\nTimeZero:%f", initial string=w152, w151, w158, w157, w156, w155, w150, w149, w148, w147, w146, w145, w144, w143, w125, w124, w123, w122, w121, w120, w119, w118, w117, w116) -> ()  [unwired: 1 in, 2 out]
        n105 = Unbundle(w141) -> ("queue out"=w133:refnum<queue>, "queue out"=w140:refnum<queue>, "queue out"=w139:refnum<queue>, "queue out"=w138:refnum<queue>, "queue out"=w137:refnum<queue>)
        n106 = for {
          tunnel: w126 -> [w313] mode=indexing
          tunnel: [w312] -> w134 mode=indexing
          tunnel: [w311] -> w135
          tunnel: w140 -> [w310]
          tunnel: w139 -> [w309]
          tunnel: w138 -> [w308]
          tunnel: w137 -> [w307]
          tunnel: "scan_selector" -> [w306]
          tunnel: w115 -> [w305]
          n107 = case shown="\"mirror\"" w306 {
            tunnel: w313 -> [w321 w348 w361 w371]
            tunnel: [w319 w336 w358 w375] -> w311
            tunnel: [w325 w337 w359 w376] -> w312
            tunnel: w310 -> [w319 _ _ _]
            tunnel: w309 -> [_ w336 _ _]
            tunnel: w308 -> [_ _ _ w375]
            tunnel: w307 -> [_ _ w358 _]
            tunnel: w305 -> [w314 w331 w355 w372]
            frame "delay", Default {
              w327 = ":" ("string")
              n108 = local read "ESP_t0"() -> (w320:dbl)
              n109 = call "time2mm.vi"("fs[1]/ps[0]"=TRUE, "Offset (mm)"=w320, "time"=w321) -> ("position (mm)"=w316:dbl)
              n110 = local read "ESP Axis"() -> (w324:i32)
              n111 = Build Array(w316) -> (w315:dbl[])
              n112 = Number To Decimal String(number=w324) -> (decimal integer string=w323:string)  [unwired: 1 in]
              n113 = Number To Fractional String(number=w316) -> (F-format string=w329:string)  [unwired: 3 in]
              n114 = call-poly <vilib>:"Write Delimited Spreadsheet.vi"("file path (dialog if empty)"=w314, "format (%.3f)"="%.6f", "1D data"=w315, "append to file? (new file:F)"=TRUE ("append to file? (F)")) -> ()  [unwired: 10 in, 2 out]
              n115 = Concatenate Strings("abs:" ("string"), w323, w327, w329, w327, "wait" ("string")) -> (w325:string)
            }
            frame "manip" {
              n116 = call-poly <vilib>:"Vector Norm.vi"("Input Vector"="scan_manip_deltas") -> ("norm"=w350:dbl)  [unwired: 9 in, 1 out]
              n117 = Divide(x="scan_manip_deltas", y=w350) -> (x/y=w349:dbl[])
              n118 = Multiply(x=w349, y=w348) -> (x*y=w334:dbl[])
              n119 = Add(x="scan_manip_start", y=w334) -> (x+y=w330:dbl[])
              n120 = call-poly <vilib>:"Write Delimited Spreadsheet.vi"("file path (dialog if empty)"=w331, "format (%.3f)"="%.6f", "1D data"=w330, "append to file? (new file:F)"=TRUE ("append to file? (F)")) -> ()  [unwired: 10 in, 2 out]
              n121 = Index Array(array=w330) -> (element #1=w339:dbl, element #2=w340:dbl, element #3=w341:dbl, element #4=w342:dbl, element #5=w343:dbl, element #6=w344:dbl)  [unwired: 6 in]
              n122 = Format Into String(format string="%g_%g_%g_%g_%g_%g", w339, w340, w341, w342, w343, w344) -> (resulting string=w346:string)  [unwired: 2 in, 1 out]
              n123 = Concatenate Strings("abs:" ("string"), w346, ":wait" ("string")) -> (w337:string)
            }
            frame "mirror" {
              n124 = call-poly <vilib>:"Vector Norm.vi"("Input Vector"="scan_mirr_deltas") -> ("norm"=w369:dbl)  [unwired: 9 in, 1 out]
              n125 = Divide(x="scan_mirr_deltas", y=w369) -> (x/y=w368:dbl[])
              n126 = Multiply(x=w368, y=w361) -> (x*y=w357:dbl[])
              n127 = Add(x="scan_mirr_start", y=w357) -> (x+y=w354:dbl[])
              n128 = call-poly <vilib>:"Write Delimited Spreadsheet.vi"("file path (dialog if empty)"=w355, "format (%.3f)"="%.6f", "1D data"=w354, "append to file? (new file:F)"=TRUE ("append to file? (F)")) -> ()  [unwired: 10 in, 2 out]
              n129 = Index Array(array=w354) -> (element #1=w364:dbl, element #2=w365:dbl)  [unwired: 2 in]
              n130 = Format Into String(format string="%g_%g", w364, w365) -> (resulting string=w367:string)  [unwired: 2 in, 1 out]
              n131 = Concatenate Strings("abs:" ("string"), w367, ":wait" ("string")) -> (w359:string)
            }
            frame "volt" {
              n132 = local read "scan_volt_parameter"() -> (w379:string)
              n133 = Build Array(w371) -> (w370:dbl[])
              n134 = Number To Fractional String(number=w371) -> (F-format string=w377:string)  [unwired: 3 in]
              n135 = Concatenate Strings("setsgl:" ("string"), w379, ":" ("string"), w377) -> (w376:string)
              n136 = call-poly <vilib>:"Write Delimited Spreadsheet.vi"("file path (dialog if empty)"=w372, "format (%.3f)"="%.6f", "1D data"=w370, "append to file? (new file:F)"=TRUE ("append to file? (F)")) -> ()  [unwired: 10 in, 2 out]
            }
          }
        }
        n137 = Build Path(base path=w132, name or relative path="RAW\\LUT.txt") -> (appended path=w130:path)
        n138 = call-poly <vilib>:"Write Delimited Spreadsheet.vi"("file path (dialog if empty)"=w130, "1D data"=string[] ["filename", "time", "delaystage", "X", "Y", "Z", "polar", "tilt", "azimuth", "mirrorX", "mirrorY", "KineticEnergy", "PassEnergy", "CoilCurrent", "WorkFunction", "DetectorVoltage", "ScreenVoltage", "ConversionVoltage", "FD1", "FD2"]) -> ("new file path (Not A Path if cancelled)"=w129:path)  [unwired: 12 in, 1 out]
        n139 = Get Date/Time In Seconds() -> (seconds since 1Jan1904=w142:timestamp)
        n140 = while {
          tunnel: w132 -> [w190]
          tunnel: w165 -> [w189]
          shift-right: [w188] -> w163
          shift-left: dbl[][][] [] -> [w187]
          tunnel: w162 -> [w186]
          tunnel: w142 -> [w185]
          tunnel: w135 -> [w184]
          tunnel: w134 -> [w183]
          tunnel: w133 -> [w182]
          shift-right: [w180] -> _
          shift-left: w129 -> [w181]
          shift-right: [w179] -> w127
          shift-left: w126 -> [w178]
          i -> [w177]
          stop <- w174 stop-if-true
          n141 = local read "meas_iter"() -> (w176:i32)
          n142 = for {
            N -> [w218]
            tunnel: w190 -> [w215]
            tunnel: w189 -> [w240]
            tunnel: w177 -> [w213]
            shift-right: [w229] -> w188
            shift-left: w187 -> [w236]
            tunnel: w186 -> [w231]
            tunnel: w185 -> [w217]
            tunnel: w184 -> [w209]
            tunnel: w183 -> [w208] mode=indexing
            tunnel: w182 -> [w207]
            shift-right: [w203] -> w180
            shift-left: w181 -> [w204]
            shift-right: [w199] -> w179
            shift-left: w178 -> [w199]
            tunnel: [w196] -> w173
            tunnel: w176 -> [w195]
            i -> [w214]
            stop <- "stop after step" stop-if-true
            n143 = Cancel Notification(0:w231) -> (11:w232:errorcluster)  [unwired: 1 in, 2 out]
            n144 = Enqueue Element(queue=w209, element=w208, error in (no error)=w232) -> (error out=w235:errorcluster)  [unwired: 1 in, 2 out]
            n145 = Equal To 0?(x=w214) -> (x = 0?=w239:bool)
            n146 = Equal To 0?(x=w213) -> (x = 0?=w238:bool)
            n147 = Get Date/Time In Seconds() -> (seconds since 1Jan1904=w205:timestamp)
            n148 = Wait on Notification(notifier=w231, error in (no error)=w235) -> (error out=w234:errorcluster)  [unwired: 2 in, 3 out]
            n149 = And(x=w239, y=w238) -> (x .and. y?=w237:bool)
            n150 = Enqueue Element(queue=w207, element="snap", error in (no error)=w234) -> (error out=w233:errorcluster)  [unwired: 1 in, 2 out]
            n151 = call "createFileStruc.vi"("i_iter"=w213, "i_delay"=w214, "meas_path"=w215) -> ("AVG file"=w210:path, "RAW file"=w201:path)  [unwired: 7 in]
            n152 = Dequeue Element(queue=w240, error in (no error)=w233) -> (element=w212:dbl[][], error out=w202:errorcluster)  [unwired: 1 in, 2 out]
            n153 = Strip Path(path=w201) -> (name=w200:string)  [unwired: 1 out]
            n154 = Array Size(array=w212) -> (size(s)=w244:i32[])
            n155 = call-poly <vilib>:"Write Delimited Spreadsheet.vi"("file path (dialog if empty)"=w201, "2D data"=w212, "error in (no error)"=w202) -> ()  [unwired: 11 in, 2 out]
            n156 = Index Array(array=w244) -> (element #1=w242:i32, element #2=w241:i32)  [unwired: 2 in]
            n157 = Subtract(x=w205, y=w217) -> (x-y=w221:dbl)
            n158 = flat-sequence {
              tunnel: "%s\\t%<%Y.%m.%d %H:%M:%S>T\\t%f\\t%f\\t%f\\t%f\\t%f\\t%f\\t%f\\t%f\\t%f\\t%f\\t%f\\t%f\\t%f\\t%f\\t%f\\t%f\\t%f\\t%f\\t%f" -> [w274]
              tunnel: w205 -> [w273]
              tunnel: w204 -> [w250]
              tunnel: [w249] -> w203
              tunnel: w202 -> [w246]
              tunnel: w200 -> [w245]
              frame #0 {
                n159 = local read "pos"() -> (w275:dbl[])
                n160 = local read "mirr_posX"() -> (w262:i32)
                n161 = local read "mirr_posY"() -> (w263:i32)
                n162 = local read "ESP_delay"() -> (w255:dbl)
                n163 = local read "phoib_I_1"() -> (w264:dbl)
                n164 = local read "phoib_I_2"() -> (w265:dbl)
                n165 = local read "phoib_I_3"() -> (w266:dbl)
                n166 = local read "phoib_I_4"() -> (w267:dbl)
                n167 = local read "phoib_I_5"() -> (w268:dbl)
                n168 = local read "phoib_I_6"() -> (w269:dbl)
                n169 = local read "phoib_I_7"() -> (w270:dbl)
                n170 = local read "phoib_I_8"() -> (w271:dbl)
                n171 = local read "phoib_I_9"() -> (w272:dbl)
                n172 = local read "ESP_pos"() -> (w254:dbl)
                n173 = Index Array(array=w275) -> (element #1=w256:dbl, element #2=w257:dbl, element #3=w258:dbl, element #4=w259:dbl, element #5=w260:dbl, element #6=w261:dbl)  [unwired: 6 in]
                n174 = Format Into String(format string=w274, error in=w246, w245, w273, w254, w255, w256, w257, w258, w259, w260, w261, w262, w263, w264, w265, w266, w267, w268, w269, w270, w271, w272) -> (resulting string=w252:string)  [unwired: 1 in, 1 out]
                n175 = Spreadsheet String To Array(format string="%s", spreadsheet string=w252, array type (2D Dbl)=string[] []) -> (array=w248:string[])  [unwired: 1 in]
                n176 = call-poly <vilib>:"Write Delimited Spreadsheet.vi"("file path (dialog if empty)"=w250, "1D data"=w248, "append to file? (new file:F)"=TRUE ("append to file? (F)")) -> ("new file path (Not A Path if cancelled)"=w249:path)  [unwired: 11 in, 1 out]
              }
            }
            n177 = case shown="True" w237 {
              tunnel: w218 -> [_ w281]
              tunnel: [w276 w279] -> w243
              tunnel: w236 -> [w276 _]
              tunnel: w242 -> [_ w278]
              tunnel: w241 -> [_ w277]
              frame False {
              }
              frame True {
                n178 = Initialize Array(0.0 ("element"), w281, w278, w277) -> (w279:dbl[][][])
              }
            }
            n179 = Increment(x=w214) -> (x+1=w225:i32)
            "current scan" <- w225
            n180 = Increment(x=w213) -> (x+1=w224:i32)
            "current iteration" <- w224
            n181 = for {
              N: w242 -> [_]
              tunnel: w214 -> [w288]
              shift-right: [w286] -> w229
              shift-left: w243 -> [w289]
              tunnel: w213 -> [w284]
              shift-right: [w283] -> w211
              shift-left: w212 -> [w285]
              tunnel: w241 -> [w282]
              i -> [w287]
              n182 = for {
                N: w282 -> [_]
                tunnel: w288 -> [w296]
                tunnel: w287 -> [w293]
                shift-right: [w295] -> w286
                shift-left: w289 -> [w297]
                tunnel: w284 -> [w291]
                shift-right: [w290] -> w283
                shift-left: w285 -> [w294]
                i -> [w292]
                n183 = in-place {
                  in-place-border: w291 -> [w303]
                  n184 = in-place-array #1(w297, w296, w293, w292) -> (w304:dbl)
                  n185 = in-place-array #2(w294, w293, w292) -> (w301:dbl)
                  n186 = Multiply(x=w304, y=w303) -> (x*y=w302:dbl)
                  n187 = Increment(x=w303) -> (x+1=w299:i32)
                  n188 = Add(x=w302, y=w301) -> (x+y=w300:dbl)
                  n189 = Divide(x=w300, y=w299) -> (x/y=w298:dbl)
                  n190 = in-place-array #1(w298) -> (w295:dbl[][][])  [unwired: 3 out]
                  n191 = in-place-array #2(w298) -> (w290:dbl[][])  [unwired: 2 out]
                }
              }
            }
            n192 = Multiply(x=w218, y=w213) -> (x*y=w220:i32)
            n193 = Multiply(x=w218, y=w195) -> (x*y=w216:i32)
            n194 = Divide(x=w225, y=w218) -> (x/y=→"scan":dbl)
            n195 = Divide(x=w224, y=w195) -> (x/y=→"iteration":dbl)
            n196 = Add(x=w214, y=w220) -> (x+y=w219:i32)
            n197 = Divide(x=w221, y=w219) -> (x/y=w191:dbl)
            n198 = Multiply(x=w191, y=w216) -> (x*y=w194:dbl)
            n199 = local write "time/step [s]"(w191) -> ()
            n200 = local write "duration [HH:MM:SS]"(w194) -> ()
            n201 = property on="mainimg" class="IntGraph (strict)"() -> ("CrsrLis"=w228:T4)  [unwired: 2 in, 2 out]
            n202 = call-poly <vilib>:"Write Delimited Spreadsheet.vi"("file path (dialog if empty)"=w210, "2D data"=w211) -> ()  [unwired: 12 in, 2 out]
            n203 = call "processData.vi"("Cursor List"=w228, "data in"=w229) -> ("Angle Chart"=→"anglegraph":dbl[][], "Energy Chart"=→"energygraph":dbl[][], "Intensity Chart"=w227:dbl[])  [unwired: 1 in]
            n204 = Bundle("Array"=w199, "Intensity Chart"=w227) -> (→"intensitygraph":cluster{"Array":dbl[], "Intensity Chart":dbl[]})  [unwired: 1 in]
            n205 = Or(x="stop after iteration", y="stop after step") -> (x .or. y?=w196:bool)
          }
          n206 = Increment(x=w177) -> (x+1=w175:i32)
          n207 = Greater Or Equal?(x=w175, y=w176) -> (x >= y?=w172:bool)
          n208 = Or(x=w173, y=w172) -> (x .or. y?=w174:bool)
        }
      }
      frame "refresh" {
        n209 = Dequeue Element(queue=w385) -> ()  [unwired: 2 in, 4 out]
        n210 = property on="mainimg" class="IntGraph (strict)"() -> ("CrsrLis"=w392:T4)  [unwired: 2 in, 2 out]
        n211 = call "processData.vi"("Cursor List"=w392, "data in"=w391) -> ("Angle Chart"=w389:dbl[][], "Energy Chart"=w390:dbl[][], "Intensity Chart"=w386:dbl[])  [unwired: 1 in]
        n212 = Bundle("Array"=w387, "Intensity Chart"=w386) -> (w388:cluster{"Array":dbl[], "Intensity Chart":dbl[]})  [unwired: 1 in]
        n213 = local write "energygraph"(w390) -> ()
        n214 = local write "intensitygraph"(w388) -> ()
        n215 = local write "anglegraph"(w389) -> ()
      }
    }
  }
  n216 = while {
    tunnel: w14 -> [w400]
    tunnel: w13 -> [w399]
    tunnel: w12 -> [w398]
    tunnel: w11 -> [w397]
    tunnel: w16 -> [w395]
    tunnel: w23 -> [w396]
    tunnel: w3 -> [w394]
    tunnel: w4 -> [w393]
    stop <- w401 stop-if-true
    n217 = event shown="[0] Timeout" {
      selector: _ -> [_ _ _ _ _ _ _ _ _ _ _ _ _ _ _ _ _ _ _ _ _ _ _ _ _ _ _ _ _]
      dyn-events: _ -> [_ _ _ _ _ _ _ _ _ _ _ _ _ _ _ _ _ _ _ _ _ _ _ _ _ _ _ _ _]
      timeout: _ -> [_ _ _ _ _ _ _ _ _ _ _ _ _ _ _ _ _ _ _ _ _ _ _ _ _ _ _ _ _]
      tunnel: [_ TRUE _ _ _ _ _ _ _ _ _ _ _ _ _ _ _ _ _ _ _ _ _ _ _ _ _ _ _] -> w401
      tunnel: w400 -> [_ w413 w426 _ _ _ _ _ w452 w454 _ _ _ _ _ _ _ _ _ _ _ _ _ _ _ _ _ _ _]
      tunnel: w399 -> [_ w412 _ w430 _ _ _ _ _ _ _ _ _ _ _ _ _ _ _ w520 _ _ w542 _ _ _ _ _ _]
      tunnel: w398 -> [_ w411 _ _ w436 _ _ _ _ _ _ _ _ _ _ _ w494 w510 w512 _ _ _ _ _ _ _ _ _ _]
      tunnel: w397 -> [_ w410 _ _ _ w442 w448 w449 _ _ _ _ _ _ _ _ _ _ _ _ _ _ _ _ _ _ _ _ _]
      tunnel: w396 -> [_ w419 _ _ _ _ _ _ _ _ _ _ _ _ _ _ _ _ _ _ _ _ _ _ _ _ _ _ _]
      tunnel: w395 -> [_ w409 _ _ _ _ _ _ _ _ w456 w458 _ _ _ _ _ _ _ _ _ _ _ _ _ _ w561 _ _]
      tunnel: w394 -> [_ w418 _ _ _ _ _ _ _ _ _ _ _ _ _ _ _ _ _ _ _ _ _ _ _ _ _ _ _]
      tunnel: w393 -> [_ w408 _ _ _ _ _ _ _ _ _ _ _ w472 _ _ _ _ _ _ _ _ _ _ _ _ _ w563 w584]
      event Timeout {
        n218 = event-data() -> ()  [unwired: 1 in, 1 out]
      }
      event "main_close": Value Change {
        w414 = "close" ("element")
        w415 = "release" ("element")
        n219 = event-data() -> ()  [unwired: 1 in, 1 out]
        n220 = Flush Queue(queue=w413) -> (queue out=w407:refnum<queue>)  [unwired: 1 in, 2 out]
        n221 = Flush Queue(queue=w412) -> (queue out=w406:refnum<queue>)  [unwired: 1 in, 2 out]
        n222 = Flush Queue(queue=w411) -> (queue out=w405:refnum<queue>)  [unwired: 1 in, 2 out]
        n223 = Flush Queue(queue=w410) -> (queue out=w404:refnum<queue>)  [unwired: 1 in, 2 out]
        n224 = Flush Queue(queue=w409) -> (queue out=w403:refnum<queue>)  [unwired: 1 in, 2 out]
        n225 = Flush Queue(queue=w408) -> (queue out=w402:refnum<queue>)  [unwired: 1 in, 2 out]
        n226 = Release Notifier(notifier=w418) -> ()  [unwired: 2 in, 3 out]
        n227 = Release Queue(queue=w419) -> ()  [unwired: 2 in, 3 out]
        n228 = Enqueue Element(queue=w407, element=w415) -> (queue out=w423:refnum<queue>)  [unwired: 2 in, 2 out]
        n229 = Enqueue Element(queue=w406, element=w415) -> (queue out=w422:refnum<queue>)  [unwired: 2 in, 2 out]
        n230 = Enqueue Element(queue=w405, element=w415) -> (queue out=w421:refnum<queue>)  [unwired: 2 in, 2 out]
        n231 = Enqueue Element(queue=w404, element=w415) -> (queue out=w420:refnum<queue>)  [unwired: 2 in, 2 out]
        n232 = Enqueue Element(queue=w402, element=w415) -> (queue out=w417:refnum<queue>, error out=w416:errorcluster)  [unwired: 2 in, 1 out]
        n233 = Enqueue Element(queue=w423, element=w414) -> ()  [unwired: 2 in, 3 out]
        n234 = Enqueue Element(queue=w422, element=w414) -> ()  [unwired: 2 in, 3 out]
        n235 = Enqueue Element(queue=w421, element=w414) -> ()  [unwired: 2 in, 3 out]
        n236 = Enqueue Element(queue=w420, element=w414) -> ()  [unwired: 2 in, 3 out]
        n237 = Enqueue Element(queue=w403, element=w414) -> ()  [unwired: 2 in, 3 out]
        n238 = Enqueue Element(queue=w417, element=w414, error in (no error)=w416) -> ()  [unwired: 1 in, 3 out]
      }
      event "cam_release", "cam_init": Value Change {
        n239 = event-data() -> ()  [unwired: 1 in, 2 out]
        n240 = Select(t="init" ("name (unnamed)"), s="cam_init", f="release" ("name (unnamed)")) -> (s? t:f=w425:string)
        n241 = Enqueue Element(queue=w426, element=w425) -> ()  [unwired: 2 in, 3 out]
      }
      event "ESP_release", "ESP_init": Value Change {
        n242 = event-data() -> ()  [unwired: 1 in, 2 out]
        n243 = Select(t="init" ("name (unnamed)"), s="ESP_init", f="release" ("name (unnamed)")) -> (s? t:f=w434:string)
        n244 = Enqueue Element(queue=w430, element=w434) -> ()  [unwired: 2 in, 3 out]
      }
      event "manip_init", "manip_release": Value Change {
        n245 = event-data() -> ()  [unwired: 1 in, 2 out]
        n246 = Flush Queue(queue=w436) -> (queue out=w435:refnum<queue>)  [unwired: 1 in, 2 out]
        n247 = Select(t="init" ("name (unnamed)"), s="manip_init", f="release" ("name (unnamed)")) -> (s? t:f=w438:string)
        n248 = Enqueue Element(queue=w435, element=w438) -> ()  [unwired: 2 in, 3 out]
      }
      event "phoib_release", "phoib_init": Value Change {
        n249 = event-data() -> ()  [unwired: 1 in, 2 out]
        n250 = Flush Queue(queue=w442) -> (queue out=w441:refnum<queue>)  [unwired: 1 in, 2 out]
        n251 = Select(t="init" ("name (unnamed)"), s="phoib_init", f="release" ("name (unnamed)")) -> (s? t:f=w444:string)
        n252 = Enqueue Element(queue=w441, element=w444) -> ()  [unwired: 2 in, 3 out]
      }
      event "phoib_standby": Value Change {
        n253 = event-data() -> ()  [unwired: 1 in, 2 out]
        n254 = Enqueue Element(queue=w448, element="standby") -> ()  [unwired: 2 in, 3 out]
      }
      event "phoib_set": Value Change {
        n255 = event-data() -> ()  [unwired: 1 in, 2 out]
        n256 = Enqueue Element(queue=w449, element="set") -> ()  [unwired: 2 in, 3 out]
      }
      event "cam_dark": Value Change {
        n257 = event-data() -> ()  [unwired: 1 in, 2 out]
        n258 = Enqueue Element(queue=w452, element="dark") -> ()  [unwired: 2 in, 3 out]
      }
      event "ROI Left", "ROI Right", "ROI Top", "ROI Bottom", "cam_exp", "binning", "gain": Value Change {
        n259 = event-data() -> ()  [unwired: 1 in, 1 out]
        n260 = Enqueue Element(queue=w454, element="set") -> ()  [unwired: 2 in, 3 out]
      }
      event "cam_saveimg": Value Change {
        n261 = event-data() -> ()  [unwired: 1 in, 1 out]
        n262 = Enqueue Element(queue=w456, element="single") -> ()  [unwired: 2 in, 3 out]
      }
      event "scan_go": Value Change {
        n263 = event-data() -> ()  [unwired: 1 in, 1 out]
        n264 = Enqueue Element(queue=w458, element="scan") -> ()  [unwired: 2 in, 3 out]
      }
      event "meas_iter", "waypoints": Value Change {
        n265 = event-data() -> ()  [unwired: 1 in, 6 out]
        n266 = local read "waypoints"() -> (w470:string[][])
        n267 = local read "meas_iter"() -> (w464:i32)
        n268 = local read "binning"() -> (w467:u16)
        n269 = call "create scan vectr.vi"("Table Control"=w470) -> ("Array"=w469:dbl[])
        n270 = Index Array(array=dbl[] [8.79, 2.2, 0.553, 0.138], index=w467) -> (element=w463:dbl)
        n271 = Array Size(array=w469) -> (size(s)=w466:i32)
        "measpoints" <- w466
        n272 = Multiply(x=w466, y=w464) -> (x*y=w461:i32)
        "total steps" <- w461
        n273 = Multiply(x=w461, y="time/step [s]") -> (x*y=→"duration [HH:MM:SS]":dbl)
        n274 = Multiply(x=w466, y=w463) -> (x*y=→"RAM [MB]":dbl)
        n275 = Multiply(x=w461, y=w463) -> (x*y=→"disk [MB]":dbl)
      }
      event "mirr_go": Value Change {
        n276 = event-data() -> ()  [unwired: 1 in, 1 out]
        n277 = Index Array(array="mirr_dest") -> (element #1=w477:i32, element #2=w476:i32)  [unwired: 2 in]
        n278 = Format Into String(format string="%g_%g", w477, w476) -> (resulting string=w474:string)  [unwired: 2 in, 1 out]
        n279 = Concatenate Strings("abs:" ("string"), w474) -> (w471:string)
        n280 = Enqueue Element(queue=w472, element=w471) -> ()  [unwired: 2 in, 3 out]
      }
      event "scan_manip_setstart": Value Change {
        n281 = event-data() -> ()  [unwired: 1 in, 1 out]
        n282 = local read "pos"() -> (w479:dbl[])
        n283 = local write "scan_manip_start"(w479) -> ()
      }
      event "scan_mirr_setstart": Value Change {
        n284 = event-data() -> ()  [unwired: 1 in, 1 out]
        n285 = local read "mirr_posX"() -> (w482:i32)
        n286 = local read "mirr_posY"() -> (w481:i32)
        n287 = Build Array(w482, w481) -> (w480:i32[])
        n288 = local write "scan_mirr_start"(w480) -> ()
      }
      event "Move Abs": Value Change {
        n289 = event-data() -> ()  [unwired: 1 in, 1 out]
        n290 = Index Array(array="dest") -> (element #1=w492:dbl, element #2=w491:dbl, element #3=w490:dbl, element #4=w489:dbl, element #5=w488:dbl, element #6=w487:dbl)  [unwired: 6 in]
        n291 = Format Into String(format string="%g_%g_%g_%g_%g_%g", w492, w491, w490, w489, w488, w487) -> (resulting string=w485:string)  [unwired: 2 in, 1 out]
        n292 = Concatenate Strings("abs:" ("string"), w485) -> (w484:string)
        n293 = Enqueue Element(queue=w494, element=w484) -> ()  [unwired: 2 in, 3 out]
      }
      event "ManipRel +", "ManipRel -": Value Change {
        n294 = event-data() -> ()  [unwired: 1 in, 2 out]
        n295 = Negate(x="manip_deltas") -> (-x=w498:dbl[])
        n296 = Select(t="manip_deltas", s="ManipRel +", f=w498) -> (s? t:f=w496:dbl[])
        n297 = Index Array(array=w496) -> (element #1=w502:dbl, element #2=w503:dbl, element #3=w504:dbl, element #4=w505:dbl, element #5=w506:dbl, element #6=w507:dbl)  [unwired: 6 in]
        n298 = Format Into String(format string="%g_%g_%g_%g_%g_%g", w502, w503, w504, w505, w506, w507) -> (resulting string=w509:string)  [unwired: 2 in, 1 out]
        n299 = Concatenate Strings("rel:" ("string"), w509, ":wait" ("string")) -> (w500:string)
        n300 = Enqueue Element(queue=w510, element=w500) -> ()  [unwired: 2 in, 3 out]
      }
      event "stop manip": Value Change {
        n301 = event-data() -> ()  [unwired: 1 in, 1 out]
        n302 = Enqueue Element(queue=w512, element="stop") -> ()  [unwired: 2 in, 3 out]
      }
      event "ESP_go": Value Change {
        w514 = ":" ("string")
        n303 = event-data() -> ()  [unwired: 1 in, 1 out]
        n304 = local read "ESP Axis"() -> (w513:i32)
        n305 = Number To Decimal String(number=w513) -> (decimal integer string=w516:string)  [unwired: 1 in]
        n306 = Number To Fractional String(number="ESP_dest") -> (F-format string=w515:string)  [unwired: 3 in]
        n307 = Concatenate Strings("abs:" ("string"), w516, w514, w515, w514) -> (w519:string)
        n308 = Enqueue Element(queue=w520, element=w519) -> ()  [unwired: 2 in, 3 out]
      }
      event "ESP_set_t0": Value Change {
        n309 = event-data() -> ()  [unwired: 1 in, 1 out]
        n310 = Current VI's Path() -> (path=w531:path)
        n311 = Strip Path(path=w531) -> (stripped path=w529:path)  [unwired: 1 out]
        n312 = Strip Path(path=w529) -> (stripped path=w528:path)  [unwired: 1 out]
        n313 = local read "ESP_pos"() -> (w530:dbl)
        "ESP_t0" <- w530
        n314 = Number To Fractional String(number=w530) -> (F-format string=w523:string)  [unwired: 3 in]
        n315 = Build Path(base path=w528, name or relative path="t0.txt") -> (appended path=w525:path)
        n316 = Get Date/Time In Seconds() -> (seconds since 1Jan1904=w527:timestamp)
        n317 = Format Date/Time String(time format string (%c)="%Y.%m.%d %H:%M", seconds (now)=w527) -> (date/time string=w524:string)  [unwired: 1 in]
        n318 = Build Array(w524, w523) -> (w522:string[])
        n319 = call-poly <vilib>:"Write Delimited Spreadsheet.vi"("file path (dialog if empty)"=w525, "1D data"=w522, "append to file? (new file:F)"=TRUE ("append to file? (F)")) -> ()  [unwired: 11 in, 2 out]
      }
      event "ESP_opent0file": Value Change {
        n320 = event-data() -> ()  [unwired: 1 in, 6 out]
        n321 = Current VI's Path() -> (path=w535:path)
        n322 = Strip Path(path=w535) -> (stripped path=w534:path)  [unwired: 1 out]
        n323 = Strip Path(path=w534) -> (stripped path=w536:path)  [unwired: 1 out]
        n324 = call <vilib>:"System Exec.vi"("wait until completion? (T)"=FALSE, "working directory"=w536, "command line"="notepad t0.txt") -> ()  [unwired: 5 in, 4 out]
      }
      event "ESP_+", "ESP_-": Value Change {
        n325 = event-data() -> ()  [unwired: 1 in, 6 out]
        n326 = local read "ESP Axis"() -> (w538:i32)
        n327 = Negate(x="ESP_delta") -> (-x=w545:dbl)
        n328 = Select(t="ESP_delta", s="ESP_+", f=w545) -> (s? t:f=w543:dbl)
        n329 = Number To Decimal String(number=w538) -> (decimal integer string=w541:string)  [unwired: 1 in]
        n330 = Number To Fractional String(number=w543) -> (F-format string=w539:string)  [unwired: 3 in]
        n331 = Concatenate Strings("rel:" ("string"), w541, ":" ("string"), w539) -> (w548:string)
        n332 = Enqueue Element(queue=w542, element=w548) -> ()  [unwired: 2 in, 3 out]
      }
      event "ESP_dest": Value Change {
        n333 = event-data() -> ()  [unwired: 1 in, 6 out]
        n334 = local read "ESP_dest"() -> (w552:dbl)
        n335 = local read "ESP_t0"() -> (w551:dbl)
        n336 = call "mm2time.vi"("fs?"=TRUE ("fs[1]/ps[0]"), "Offset (mm)"=w551, "distance (mm)"=w552) -> ("time in fs/ps seconds"=w549:dbl)
        n337 = local write "ESP_dest_t"(w549) -> ()
      }
      event "ESP_dest_t": Value Change {
        n338 = event-data() -> ()  [unwired: 1 in, 1 out]
        n339 = local read "ESP_t0"() -> (w555:dbl)
        n340 = call "time2mm.vi"("fs[1]/ps[0]"=TRUE, "Offset (mm)"=w555, "time"="ESP_dest_t") -> ("position (mm)"=w553:dbl)
        n341 = local write "ESP_dest"(w553) -> ()
      }
      event "load delay table": Value Change {
        n342 = event-data() -> ()  [unwired: 1 in, 6 out]
        n343 = call-poly <vilib>:"Read Delimited Spreadsheet.vi"() -> ("all rows"=w558:string[][], "error out"=w557:errorcluster)  [unwired: 10 in, 4 out]
        n344 = case shown="No Error" w557 {
          tunnel: w558 -> [w559 _]
          frame No Error {
            n345 = local write "waypoints"(w559) -> ()
          }
          frame Error {
          }
        }
      }
      event "mainimg": Cursor Release {
        n346 = event-data() -> ()  [unwired: 1 in, 1 out]
        n347 = Enqueue Element(queue=w561, element="refresh") -> ()  [unwired: 2 in, 3 out]
      }
      event "mirr_init", "mirr_release": Value Change {
        n348 = event-data() -> ()  [unwired: 1 in, 6 out]
        n349 = Flush Queue(queue=w563) -> (queue out=w564:refnum<queue>)  [unwired: 1 in, 2 out]
        n350 = Select(t="init" ("name (unnamed)"), s="mirr_init", f="release" ("name (unnamed)")) -> (s? t:f=w565:string)
        n351 = Enqueue Element(queue=w564, element=w565) -> ()  [unwired: 2 in, 3 out]
      }
      event "mirr_X-", "mirr_X+", "mirr_Y+", "mirr_Y-": Value Change {
        n352 = event-data() -> ()  [unwired: 1 in, 1 out]
        n353 = local read "mirr_X#"() -> (w575:u8)
        n354 = local read "mirr_Y#"() -> (w574:u8)
        n355 = Or(x="mirr_X+", y="mirr_X-") -> (x .or. y?=w576:bool)
        n356 = Or(x="mirr_X-", y="mirr_Y-") -> (x .or. y?=w582:bool)
        n357 = Negate(x="mirr_rel") -> (-x=w581:i32)
        n358 = Select(t=w575, s=w576, f=w574) -> (s? t:f=w573:u8)
        n359 = Select(t=w581, s=w582, f="mirr_rel") -> (s? t:f=w570:i32)
        n360 = Number To Decimal String(number=w573) -> (decimal integer string=w572:string)  [unwired: 1 in]
        n361 = Number To Decimal String(number=w570) -> (decimal integer string=w569:string)  [unwired: 1 in]
        n362 = Concatenate Strings("rel:" ("string"), w572, ":" ("string"), w569) -> (w568:string)
        n363 = Enqueue Element(queue=w584, element=w568) -> ()  [unwired: 2 in, 3 out]
      }
    }
  }
  n364 = while {
    tunnel: w14 -> [w611]
    shift-right: [w605] -> _
    shift-left: _ -> [w604]
    shift-right: [w603] -> _
    shift-left: _ -> [w601]
    shift-right: [w602] -> _
    shift-left: _ -> [w600]
    shift-right: [w597] -> _
    shift-left: 0 -> [w598]
    shift-right: [w596] -> _
    shift-left: _ -> [w595]
    shift-right: [w594] -> _
    shift-left: _ -> [w593]
    tunnel: w23 -> [w592]
    shift-right: [w591] -> _
    shift-left: _ -> [w590]
    shift-right: [w588] -> _
    shift-left: _ -> [w587]
    shift-right: [w586] -> _
    shift-left: _ -> [w585]
    i -> [w589]
    stop <- w599 stop-if-true
    # "cam"
    n365 = Preview Queue Element(queue=w611, timeout in ms (-1)=w598) -> (queue out=w610:refnum<queue>, element=w609:string)  [unwired: 1 in, 2 out]
    n366 = Match Pattern(string=w609, regular expression=":") -> (before substring=w606:string, after substring=w607:string)  [unwired: 1 in, 2 out]
    n367 = case shown="\"init\"" w606 {
      tunnel: w610 -> [w623 w655 w688 w701 _ w789 w819 w884]
      tunnel: w607 -> [_ _ _ _ _ _ _ _]
      tunnel: [w617 w642 w687 w699 w742 w786 w804 w882] -> w605
      tunnel: w604 -> [_ _ w687 w699 w742 w786 w804 w882]
      tunnel: [w622 w656 u64 0 ("Hout") w698 w746 w787 w814 w881] -> w603
      tunnel: [w624 w657 w684 w697 w747 w788 w805 w880] -> w602
      tunnel: w601 -> [_ w659 w686 w698 w749 w791 w816 w881]
      tunnel: w600 -> [_ w658 _ w697 w748 w790 w815 w880]
      tunnel: [_ _ _ TRUE _ _ _ _] -> w599
      tunnel: [_ _ -1 _ _ _ _ -1] -> w597
      tunnel: [w616 w643 _ _ w756 _ _ _] -> w596
      tunnel: w595 -> [w616 w643 _ _ w755 _ _ _]
      tunnel: [w617 w645 w682 w696 w751 w780 w817 w879] -> w594
      tunnel: w593 -> [_ w645 w682 w696 w751 _ w817 w879]
      tunnel: w592 -> [_ _ _ _ _ _ w808 _]
      tunnel: [w614 w640 w681 w694 w709 w777 w811 w878] -> w591
      tunnel: w590 -> [w614 w640 w681 w694 w744 w777 w811 w878]
      tunnel: w589 -> [_ _ _ _ w717 _ _ _]
      tunnel: [w615 w641 w680 w695 w743 w776 w810 w877] -> w588
      tunnel: w587 -> [w615 w641 w680 w695 w716 w776 w810 w877]
      tunnel: [w613 w637 refnum<k21> refnum ("task out") w693 w702 w775 w801 w876] -> w586
      tunnel: w585 -> [_ w637 w679 w693 w702 w775 w802 w876]
      frame "init" {
        w617 = u16[][] []
        n368 = flat-sequence {
          tunnel: [w626] -> w621
          tunnel: [w627] -> w620
          tunnel: [w635] -> w622
          tunnel: [w636] -> w624
          tunnel: w621 -> [w636]
          tunnel: w620 -> [w635]
          frame #0 {
            n369 = local write "cam_con?"(FALSE ("cam_con?")) -> ()
          }
          frame #1 {
            n370 = call "SCInitBoard.vi"("boardnr"="board number") -> ("Hout"=w630:u32, "error out"=w631:errorcluster)  [unwired: 1 in, 1 out]
            n371 = call "SCSetupCamera.vi"("Handle"=w630, "error in (no error)"=w631) -> ("Hout"=w632:u64, "error out"=w633:errorcluster)  [unwired: 1 out]
            n372 = call "SCStopCOC.vi"("error in (no error)"=w633, "Stop mode"=0, "Handle"=w632) -> ("error out"=w626:errorcluster, "Hout"=w627:u64)
          }
          frame #2 {
            n373 = local write "cam_con?"(TRUE ("cam_con?")) -> ()
          }
        }
        n374 = Dequeue Element(queue=w623) -> (queue out=w619:refnum<queue>)  [unwired: 2 in, 3 out]
        n375 = Enqueue Element At Opposite End(queue=w619, element="set") -> ()  [unwired: 2 in, 3 out]
        n376 = call-poly <vilib>:"DAQmx Create Virtual Channel.vi"("lines"=tag "Dev3/port0/line0") -> ("task out"=w613:refnum<k21>)  [unwired: 13 in, 1 out]
      }
      frame "set" {
        n377 = Dequeue Element(queue=w655) -> ()  [unwired: 2 in, 4 out]
        n378 = call "SCStopCOC.vi"("error in (no error)"=w658, "Stop mode"=0, "Handle"=w659) -> ("error out"=w674:errorcluster, "Hout"=w673:u64)
        n379 = Bundle By Name(cluster=cluster{"Delay":dbl, "Exposure ":dbl} {"Delay"=0.0, "Exposure "=0.0} ("Delay and exposure"), "Exposure"="cam_exp") -> (w652:cluster{"Delay":dbl, "Exposure ":dbl})
        n380 = Bundle By Name(cluster=T5 {"Camera type"=0, "Operating mode\nHP & QE / HS & DiCam Pro "=0, "Frame trigger \n(High Performance and QE only)"=0, "Sequence trigger"=0, "Low Light\n(QE only)"=FALSE, "Gain"=FALSE, "Horzontal\nbinning"=0, "Vertical\nbinning "=0, "ROI Left"=1, "ROI Right"=20, "ROI Top"=1, "ROI Bottom"=15} ("Camera controls"), "Operating mode\nHP & QE / HS & DiCam Pro"="Operating mode\nHP & QE / HS & DiCam Pro", "Horzontal\nbinning"="binning", "Vertical\nbinning"="binning", "ROI Left"="ROI Left", "ROI Right"="ROI Right", "ROI Top"="ROI Top", "ROI Bottom"="ROI Bottom", "Gain"="gain", "Frame trigger \n(High Performance and QE only)"="Frame trigger \n(High Performance and QE only)") -> (w669:T5)
        n381 = call "New delay and exposure forma.vi"("Operating mode\nHP & QE / HS & DiCam Pro"="Operating mode\nHP & QE / HS & DiCam Pro", "Delay and exposure"=w652) -> ("Output table"=w670:string)  [unwired: 3 in]
        n382 = call "SCSetCoC.vi"("error in (no error)"=w674, "Delay and exposure table"=w670, "Camera controls"=w669, "Handle"=w673) -> ("error out"=w662:errorcluster, "Hout"=w661:u64)  [unwired: 1 out]
        n383 = call "SCGetImageSize.vi"("Handle"=w661, "error in (no error)"=w662) -> ("Hout"=w660:u64, "error out"=w644:errorcluster, "Horizontal size"=w649:i32, "Vertical size"=w648:i32)  [unwired: 2 out]
        n384 = Greater?(x=w649, y=w648) -> (0:w650:bool)
        n385 = Initialize Array(u16 0 ("dimension size"), w648, w649) -> (w642:u16[][])
        n386 = call "SCRun.vi"("error in (no error)"=w644, "Run mode"=0, "Handle"=w660) -> ("error out"=w657:errorcluster, "Hout"=w656:u64)  [unwired: 1 out]
        n387 = Select(t=w649, s=w650, f=w648) -> (s? t:f=w647:i32)
        n388 = property on="mainimg" class="IntGraph (strict)"("XScale.Maximum"=w647, "YScale.Maximum"=w647) -> ()  [unwired: 2 in, 2 out]
      }
      frame "release" {
        n389 = Dequeue Element(queue=w688) -> (queue out=w675:refnum<queue>)  [unwired: 2 in, 3 out]
        n390 = flat-sequence {
          tunnel: w686 -> [w690]
          tunnel: [w689] -> w683
          tunnel: [w692] -> w684
          tunnel: w683 -> [w692]
          frame #0 {
            n391 = call "SCCloseBoard.vi"("Handle"=w690) -> ("error out"=w689:errorcluster)  [unwired: 1 in, 2 out]
          }
          frame #1 {
            n392 = local write "cam_con?"(FALSE ("cam_con?")) -> ()
          }
        }
        n393 = Enqueue Element(queue=w675, element="suspend") -> ()  [unwired: 2 in, 3 out]
        n394 = call <vilib>:"DAQmx Clear Task.vi"("task in"=w679) -> ()  [unwired: 14 in, 1 out]
      }
      frame "close" {
        n395 = Release Queue(queue=w701) -> ()  [unwired: 2 in, 3 out]
      }
      frame "idle", Default {
        n396 = call "grabimg.vi"("array in"=w742, "error in"=w748, "Hin"=w749) -> ("error out"=w747:errorcluster, "imgdata"=w745:i32[][], "Hout"=w746:u64)  [unwired: 6 in]
        n397 = local read "lower threshold"() -> (w740:i32)
        n398 = case shown="False" "cam_dark?" {
          tunnel: w751 -> [_ w774]
          tunnel: [w771 w773] -> w741
          tunnel: w745 -> [w771 w772]
          frame False {
          }
          frame True {
            n399 = Subtract(x=w772, y=w774) -> (x-y=w773:dbl[][])
          }
        }
        n400 = call "filtr_b.vi"("threshold"=w740, "input array"=w741) -> ("output array"=w732:dbl[][])  [unwired: 9 in]
        n401 = call <vilib>:"High Resolution Relative Seconds.vi"() -> ("relative seconds"=w756:dbl)
        n402 = Subtract(x=w756, y=w755) -> (x-y=w754:dbl)
        n403 = Array Size(array=w732) -> (size(s)=w731:i32[])
        n404 = Reciprocal(x=w754) -> (1/x=→"cam_fps":dbl)
        n405 = Index Array(array=w731) -> (element #1=w726:i32, element #2=w725:i32)  [unwired: 2 in]
        n406 = Subtract(x=w717, y=w716) -> (x-y=w715:i32)
        n407 = Less Or Equal?(x="pics2avg", y=w715) -> (x <= y?=w738:bool)
        n408 = And(x="reset every n pics", y=w738) -> (x .and. y?=w736:bool)
        n409 = Not(x=w736) -> (.not. x?=w735:bool)
        n410 = call-poly <vilib>:"Ramp Pattern.vi"("start"=0.0, "end"=w726, "samples"=w726) -> ("Ramp Pattern"=w721:dbl[])  [unwired: 7 in, 1 out]
        n411 = call-poly <vilib>:"Ramp Pattern.vi"("start"=0.0, "end"=w725, "samples"=w725) -> ("Ramp Pattern"=w722:dbl[])  [unwired: 7 in, 1 out]
        n412 = property on="mainimg" class="IntGraph (strict)"() -> ("CrsrLis"=w714:T4)  [unwired: 2 in, 2 out]
        n413 = And(x="cam_liveavg", y=w735) -> (x .and. y?=w733:bool)
        n414 = case shown="False" w733 {
          tunnel: w732 -> [w761 w767]
          tunnel: [w761 w764] -> w709
          tunnel: w744 -> [_ w769]
          tunnel: w717 -> [w762 _]
          tunnel: [w762 w770] -> w743
          tunnel: w716 -> [_ w770]
          tunnel: w715 -> [_ w763]
          frame False {
          }
          frame True {
            n415 = Multiply(x=w769, y=w763) -> (x*y=w768:dbl[][])
            n416 = Increment(x=w763) -> (x+1=w765:i32)
            n417 = Add(x=w768, y=w767) -> (x+y=w766:dbl[][])
            n418 = Divide(x=w766, y=w765) -> (x/y=w764:dbl[][])
          }
        }
        "mainimg" <- w709
        n419 = Index Array(array=w714) -> (element #1=w712:T6, element #2=w713:T6)  [unwired: 2 in]
        n420 = Unbundle By Name(w712) -> ("Position.X"=w706:dbl, "Position.Y"=w708:dbl)
        n421 = Unbundle By Name(w713) -> ("Position.X"=w710:dbl, "Position.Y"=w711:dbl)
        n422 = Array Max & Min(array=w709) -> (max value=→"max":dbl)  [unwired: 3 out]
        n423 = Subtract(x=w711, y=w708) -> (x-y=w707:dbl)
        n424 = Subtract(x=w710, y=w706) -> (x-y=w705:dbl)
        n425 = Array Subset(array=w709, index (row)=w708, length (row)=w707) -> (w720:dbl[][])  [unwired: 2 in]
        n426 = Array Subset(array=w709, index (col)=w706, length (col)=w705) -> (w718:dbl[][])  [unwired: 2 in]
        n427 = Array Subset(array=w709, index (row)=w708, length (row)=w707, index (col)=w706, length (col)=w705) -> (w704:dbl[][])
        n428 = Transpose 2D Array(2D array=w720) -> (transposed array=w719:dbl[][])
        n429 = Add Array Elements(numeric array=w704) -> (sum=→"sum" →"Waveform Chart":dbl)
        n430 = for {
          tunnel: w718 -> [w758] mode=indexing
          tunnel: [w757] -> w728 mode=indexing
          n431 = Add Array Elements(numeric array=w758) -> (sum=w757:dbl)
        }
        n432 = for {
          tunnel: w719 -> [w760] mode=indexing
          tunnel: [w759] -> w727 mode=indexing
          n433 = Add Array Elements(numeric array=w760) -> (sum=w759:dbl)
        }
        n434 = Bundle("Ramp Pattern"=w722, w727) -> (→"G2 X":cluster{"Ramp Pattern":dbl[], dbl[]})  [unwired: 1 in]
        n435 = Bundle(w728, "Ramp Pattern"=w721) -> (→"G2 Y":cluster{dbl[], "Ramp Pattern":dbl[]})  [unwired: 1 in]
      }
      frame "dark" {
        n436 = Dequeue Element(queue=w789) -> ()  [unwired: 2 in, 4 out]
        n437 = Array Size(array=w786) -> (size(s)=w785:i32[])
        n438 = Index Array(array=w785) -> (element #1=w784:i32, element #2=w783:i32)  [unwired: 2 in]
        n439 = Initialize Array(0.0 ("element"), w784, w783) -> (w781:dbl[][])
        n440 = for {
          N: "dark avg" -> [_]
          tunnel: w791 -> [w799]
          tunnel: w790 -> [w798]
          tunnel: [w797] -> w788
          tunnel: w786 -> [w796]
          tunnel: [w795] -> w787
          shift-right: [w792] -> w779
          shift-left: w781 -> [w793]
          n441 = call "grabimg.vi"("array in"=w796, "error in"=w798, "Hin"=w799) -> ("error out"=w797:errorcluster, "imgdata"=w794:i32[][], "Hout"=w795:u64)  [unwired: 6 in]
          n442 = Add(x=w794, y=w793) -> (x+y=w792:dbl[][])
        }
        n443 = Divide(x=w779, y="dark avg") -> (x/y=w780:dbl[][])
      }
      frame "snap" {
        n444 = Dequeue Element(queue=w819) -> ()  [unwired: 2 in, 4 out]
        n445 = local read "cam_dark?"() -> (w818:bool)
        n446 = local read "cam_avgs"() -> (w813:i32)
        n447 = To Double Precision Float(number=w804) -> (double precision float=w803:dbl[][])
        n448 = Equal To 0?(x="aq.mode") -> (x = 0?=w806:bool)
        n449 = Get Date/Time In Seconds() -> (seconds since 1Jan1904=w809:timestamp)
        n450 = for {
          N: w813 -> [w831]
          shift-right: [w848] -> w814
          shift-left: w816 -> [w850]
          shift-right: [w836] -> w812
          shift-left: w815 -> [w849]
          tunnel: w818 -> [w846]
          tunnel: w817 -> [w845]
          tunnel: w804 -> [w844]
          tunnel: w809 -> [w840]
          tunnel: w806 -> [w824]
          shift-right: [w832] -> w800
          shift-left: w803 -> [w833]
          shift-right: [w822] -> w801
          shift-left: w802 -> [w822]
          i -> [w820]
          stop <- "abort acq." stop-if-true
          n451 = call "grabimg.vi"("array in"=w844, "error in"=w849, "Hin"=w850) -> ("error out"=w836:errorcluster, "imgdata"=w847:i32[][], "Hout"=w848:u64)  [unwired: 6 in]
          n452 = local read "lower threshold"() -> (w827:i32)
          n453 = Increment(x=w820) -> (x+1=w829:i32)
          "acq. imgs" <- w829
          n454 = Get Date/Time In Seconds() -> (seconds since 1Jan1904=w843:timestamp)
          n455 = case shown="True" w846 {
            tunnel: w847 -> [w872 w875]
            tunnel: w845 -> [_ w874]
            tunnel: [w872 w873] -> w826
            frame False {
            }
            frame True {
              n456 = Subtract(x=w875, y=w874) -> (x-y=w873:dbl[][])
            }
          }
          n457 = Divide(x=w829, y=w831) -> (x/y=→"snap_prog":dbl)
          n458 = Subtract(x=w843, y=w840) -> (x-y=w842:dbl)
          n459 = call "filtr_b.vi"("threshold"=w827, "input array"=w826) -> ("output array"=w825:dbl[][])  [unwired: 9 in]
          n460 = Divide(x=w842, y=w820) -> (x/y=w838:dbl)
          n461 = Multiply(x=w838, y=w831) -> (x*y=w841:dbl)
          n462 = Reciprocal(x=w838) -> (1/x=w837:dbl)
          n463 = case shown="True" "count?" {
            tunnel: w825 -> [w863 w865]
            tunnel: "e-size" -> [_ w867]
            tunnel: w827 -> [_ w866]
            tunnel: [w863 w864] -> w823
            frame False {
            }
            frame True {
              n464 = Array Size(array=w865) -> (size(s)=w869:i32[])
              n465 = call "findr.vi"("thresh"=w866, "esize"=w867, "inp array"=w865) -> ("locs"=w868:i32[][])  [unwired: 8 in]
              n466 = Index Array(array=w869) -> (element #1=w871:i32, element #2=w870:i32)  [unwired: 2 in]
              n467 = call "drawe.vi"("Ysize"=w871, "Xsize"=w870, "pos array"=w868) -> ("img out"=w864:i32[][])  [unwired: 8 in]
            }
          }
          n468 = Add(x=w841, y=w840) -> (x+y=→"ETA":timestamp)
          n469 = local write "cam_fps"(w837) -> ()
          n470 = local write "mainimg"(w825) -> ()
          n471 = case shown="True" w824 {
            tunnel: w823 -> [w853 w861]
            tunnel: w833 -> [w855 w860]
            tunnel: [w854 w858] -> w832
            tunnel: [w852 w857] -> w821
            tunnel: w820 -> [w851 w856]
            frame False {
              n472 = Add(x=w853, y=w855) -> (x+y=w854:dbl[][])
              n473 = Increment(x=w851) -> (x+1=w852:i32)
            }
            frame True {
              n474 = Multiply(x=w860, y=w856) -> (x*y=w862:dbl[][])
              n475 = Increment(x=w856) -> (x+1=w857:i32)
              n476 = Add(x=w861, y=w862) -> (x+y=w859:dbl[][])
              n477 = Divide(x=w859, y=w857) -> (x/y=w858:dbl[][])
            }
          }
          "Pics L" <- w821
          n478 = local write "sideimg"(w832) -> ()
        }
        n479 = Enqueue Element(queue=w808, element=w800, error in (no error)=w812) -> (error out=w805:errorcluster)  [unwired: 1 in, 2 out]
      }
      frame "suspend" {
        n480 = Dequeue Element(queue=w884) -> ()  [unwired: 2 in, 4 out]
      }
    }
    "cam_error" <- w602
  }
  n481 = while {
    tunnel: w4 -> [w893]
    shift-right: [w890] -> _
    shift-left: _ -> [w891]
    tunnel: w3 -> [w889]
    shift-right: [w888] -> _
    shift-left: _ -> [w887]
    shift-right: [w885] -> _
    shift-left: _ -> [w886]
    stop <- w892 stop-if-true
    # "mirr"
    n482 = Preview Queue Element(queue=w893, timeout in ms (-1)=w891) -> (queue out=w896:refnum<queue>, element=w897:string)  [unwired: 1 in, 2 out]
    n483 = Match Pattern(string=w897, regular expression=":") -> (before substring=w895:string, after substring=w894:string)  [unwired: 1 in, 2 out]
    n484 = case shown="\"init\"" w895 {
      tunnel: w896 -> [w932 w942 w957 w961 w964 w969 _]
      tunnel: w894 -> [w926 w943 _ _ _ _ _]
      tunnel: [_ _ _ TRUE _ _ _] -> w892
      tunnel: [_ _ _ _ -1 _ _] -> w890
      tunnel: w889 -> [w899 _ _ _ _ _ _]
      tunnel: [w918 w939 refnum<visa-resource-name> refnum ("VISA resource name out") w959 w963 w968 w974] -> w888
      tunnel: w887 -> [w931 w941 w956 w959 w963 _ w978]
      tunnel: [w903 w938 w955 w958 w962 w967 w973] -> w885
      tunnel: w886 -> [w930 w940 _ w958 w962 _ w977]
      frame "abs" {
        w914 = u8 20 items=["Echo"=55, "Home"=1, "Move Absolute"=20, "Move Relative"=21, "Move at Constant Speed"=22, "Renumber"=2, "Restore Settings"=36, "Stop"=23] ("Command")
        w929 = u8 20 items=["Echo"=55, "Home"=1, "Move Absolute"=20, "Move Relative"=21, "Move at Constant Speed"=22, "Renumber"=2, "Restore Settings"=36, "Stop"=23] ("Command")
        n485 = Dequeue Element(queue=w932) -> ()  [unwired: 2 in, 4 out]
        n486 = Match Pattern(string=w926, regular expression=":") -> (before substring=w916:string, after substring=w902:string)  [unwired: 1 in, 2 out]
        n487 = Equal?(x=w902, y="wait") -> (x = y?=w900:bool)
        n488 = Scan From String(format string="%g_%g", input string=w916) -> (output 1=w911:dbl, output 2=w910:dbl)  [unwired: 4 in, 3 out]
        n489 = local read "mirr_X#"() -> (w913:u8)
        n490 = Bundle("mirr_X#"=w913, "Command"=w929, w911, "Response Count"=1) -> (w925:T7)  [unwired: 1 in]
        n491 = local read "mirr_Y#"() -> (w912:u8)
        n492 = call "Request Command.vi"("error in (no error)"=w930, "Request"=w925, "VISA resource name"=w931) -> ("error out"=w907:errorcluster, "VISA resource name out"=w908:refnum<visa-resource-name>)  [unwired: 5 in, 2 out]
        n493 = Bundle("mirr_Y#"=w912, "Command"=w914, w910, "Response Count"=1) -> (w909:T8)  [unwired: 1 in]
        n494 = call "Request Command.vi"("error in (no error)"=w907, "Request"=w909, "VISA resource name"=w908) -> ("error out"=w905:errorcluster, "VISA resource name out"=w906:refnum<visa-resource-name>)  [unwired: 5 in, 2 out]
        n495 = local read "mirr_X#"() -> (w923:u8)
        n496 = call "zaber_readpos.vi"("error in (no error)"=w905, "axis"=w923, "VISA in"=w906) -> ("error out"=w919:errorcluster, "position"=w924:i32, "VISA out"=w920:refnum<visa-resource-name>)  [unwired: 6 in]
        n497 = local read "mirr_Y#"() -> (w921:u8)
        n498 = local write "mirr_posX"(w924) -> ()
        n499 = call "zaber_readpos.vi"("error in (no error)"=w919, "axis"=w921, "VISA in"=w920) -> ("error out"=w904:errorcluster, "position"=w922:i32, "VISA out"=w918:refnum<visa-resource-name>)  [unwired: 6 in]
        n500 = local write "mirr_posY"(w922) -> ()
        n501 = case shown="True" w900 {
          tunnel: w904 -> [w933 w937]
          tunnel: [w933 w936] -> w903
          tunnel: w899 -> [_ w935]
          frame False {
          }
          frame True {
            n502 = Send Notification(notification=TRUE, notifier=w935, error in (no error)=w937) -> (error out=w936:errorcluster)  [unwired: 1 out]
          }
        }
      }
      frame "rel" {
        w946 = u8 21 items=["Echo"=55, "Home"=1, "Move Absolute"=20, "Move Relative"=21, "Move at Constant Speed"=22, "Renumber"=2, "Restore Settings"=36, "Stop"=23] ("Command")
        n503 = Dequeue Element(queue=w942) -> ()  [unwired: 2 in, 4 out]
        n504 = Match Pattern(string=w943, regular expression=":") -> (before substring=w948:string, after substring=w947:string)  [unwired: 1 in, 2 out]
        n505 = Decimal String To Number(string=w948) -> (number=w950:i32)  [unwired: 2 in, 1 out]
        n506 = Decimal String To Number(string=w947) -> (number=w951:i32)  [unwired: 2 in, 1 out]
        n507 = Bundle(w950, "Command"=w946, w951, "Response Count"=1) -> (w944:T9)  [unwired: 1 in]
        n508 = call "Request Command.vi"("error in (no error)"=w940, "Request"=w944, "VISA resource name"=w941) -> ("error out"=w938:errorcluster, "VISA resource name out"=w939:refnum<visa-resource-name>)  [unwired: 5 in, 2 out]
      }
      frame "release" {
        n509 = Dequeue Element(queue=w957) -> (queue out=w953:refnum<queue>)  [unwired: 2 in, 3 out]
        n510 = Enqueue Element(queue=w953, element="suspend") -> ()  [unwired: 2 in, 3 out]
        n511 = call "Close.vi"("VISA resource name"=w956) -> ("error out"=w955:errorcluster)  [unwired: 9 in, 1 out]
      }
      frame "close" {
        n512 = Release Queue(queue=w961) -> ()  [unwired: 2 in, 3 out]
      }
      frame "suspend" {
        n513 = Dequeue Element(queue=w964) -> ()  [unwired: 2 in, 4 out]
      }
      frame "init" {
        n514 = Dequeue Element(queue=w969) -> ()  [unwired: 2 in, 4 out]
        n515 = call "Initialize.vi"("VISA resource name"="mirr_VISA") -> ("error out"=w967:errorcluster, "VISA resource name out"=w968:refnum<visa-resource-name>)  [unwired: 8 in, 1 out]
      }
      frame "idle", Default {
        n516 = local read "mirr_X#"() -> (w979:u8)
        n517 = call "zaber_readpos.vi"("error in (no error)"=w977, "axis"=w979, "VISA in"=w978) -> ("error out"=w975:errorcluster, "position"=→"mirr_posX":i32, "VISA out"=w976:refnum<visa-resource-name>)  [unwired: 6 in]
        n518 = local read "mirr_Y#"() -> (w972:u8)
        n519 = call "zaber_readpos.vi"("error in (no error)"=w975, "axis"=w972, "VISA in"=w976) -> ("error out"=w973:errorcluster, "position"=→"mirr_posY":i32, "VISA out"=w974:refnum<visa-resource-name>)  [unwired: 6 in]
      }
    }
    "mirr_Error" <- w885
  }
  n520 = while {
    tunnel: w13 -> [w988]
    shift-right: [w986] -> _
    shift-left: _ -> [w984]
    shift-right: [w985] -> _
    shift-left: _ -> [w983]
    shift-right: [w981] -> _
    shift-left: 0 -> [w982]
    tunnel: w3 -> [w980]
    stop <- w987 stop-if-true
    # "ESP"
    n521 = Preview Queue Element(queue=w988, timeout in ms (-1)=w982) -> (queue out=w991:refnum<queue>, element=w992:string)  [unwired: 1 in, 2 out]
    n522 = Match Pattern(string=w992, regular expression=":") -> (before substring=w990:string, after substring=w989:string)  [unwired: 1 in, 2 out]
    n523 = case shown="\"init\"" w990 {
      tunnel: w991 -> [_ w1003 w1021 w1063 w1066 w1073 w1078]
      tunnel: w989 -> [_ w1008 w1028 _ _ _ _]
      tunnel: [_ _ _ _ _ TRUE _] -> w987
      tunnel: [w995 w1010 w1022 w1061 refnum<visa-resource-name> refnum ("VISA resource name out") w1070 w1077] -> w986
      tunnel: [w994 w1011 w1020 w1060 w1068 w1071 w1076] -> w985
      tunnel: w984 -> [w999 w1013 w1026 w1061 w1069 w1070 _]
      tunnel: w983 -> [w998 w1012 w1027 w1060 _ w1071 _]
      tunnel: [_ _ _ -1 _ _ _] -> w981
      tunnel: w980 -> [_ _ w1014 _ _ _ _]
      frame "idle", Default {
        n524 = local read "ESP Axis"() -> (w996:i32)
        n525 = local read "ESP_t0"() -> (w1002:dbl)
        n526 = call "Read Actual Position.vi"("error in (no error)"=w998, "Axis (1)"=w996, "VISA resource name"=w999) -> ("error out"=w994:errorcluster, "Position (units)"=w997:dbl, "VISA resource name out"=w995:refnum<visa-resource-name>)  [unwired: 2 in]
        "ESP_pos" <- w997
        n527 = call "mm2time.vi"("fs?"=TRUE, "Offset (mm)"=w1002, "distance (mm)"=w997) -> ("time in fs/ps seconds"=→"ESP_delay":dbl)
      }
      frame "rel" {
        n528 = Match Pattern(string=w1008, regular expression=":") -> (before substring=w1007:string, after substring=w1006:string)  [unwired: 1 in, 2 out]
        n529 = Dequeue Element(queue=w1003) -> ()  [unwired: 2 in, 4 out]
        n530 = Decimal String To Number(string=w1007) -> (number=w1005:i32)  [unwired: 2 in, 1 out]
        n531 = Fract/Exp String To Number(string=w1006) -> (number=w1004:dbl)  [unwired: 3 in, 1 out]
        n532 = call "Move Relative.vi"("error in (no error)"=w1012, "Position (0 units)"=w1004, "Axis (1)"=w1005, "VISA resource name"=w1013) -> ("error out"=w1011:errorcluster, "VISA resource name out"=w1010:refnum<visa-resource-name>)  [unwired: 2 in]
      }
      frame "abs" {
        n533 = Dequeue Element(queue=w1021) -> ()  [unwired: 2 in, 4 out]
        n534 = Match Pattern(string=w1028, regular expression=":") -> (before substring=w1029:string, after substring=w1018:string)  [unwired: 1 in, 2 out]
        n535 = Match Pattern(string=w1018, regular expression=":") -> (before substring=w1017:string, after substring=w1016:string)  [unwired: 1 in, 2 out]
        n536 = Decimal String To Number(string=w1029) -> (number=w1025:i32)  [unwired: 2 in, 1 out]
        n537 = Fract/Exp String To Number(string=w1017) -> (number=w1015:dbl)  [unwired: 3 in, 1 out]
        n538 = call "Move Absolute.vi"("error in (no error)"=w1027, "Position (0 units)"=w1015, "Axis (1)"=w1025, "VISA resource name"=w1026) -> ("error out"=w1023:errorcluster, "VISA resource name out"=w1024:refnum<visa-resource-name>)  [unwired: 2 in]
        n539 = case shown="\"wait\"" w1016 {
          tunnel: w1025 -> [_ w1048]
          tunnel: w1024 -> [w1032 w1050]
          tunnel: w1023 -> [w1031 w1049]
          tunnel: [w1032 w1037] -> w1022
          tunnel: [w1031 w1045] -> w1020
          tunnel: w1014 -> [_ w1044]
          frame "", Default {
          }
          frame "wait" {
            n540 = while {
              tunnel: w1048 -> [w1059]
              shift-right: [w1056] -> w1047
              shift-left: w1050 -> [w1058]
              shift-right: [w1055] -> w1046
              shift-left: w1049 -> [w1057]
              stop <- w1054 stop-if-true
              n541 = call "Get Axis Motion Status.vi"("error in (no error)"=w1057, "Axis (1)"=w1059, "VISA resource name"=w1058) -> ("error out"=w1055:errorcluster, "Motion Done"=w1054:bool, "VISA resource name out"=w1056:refnum<visa-resource-name>)  [unwired: 2 in]
            }
            n542 = flat-sequence {
              tunnel: w1047 -> [w1053]
              tunnel: w1046 -> [w1052]
              tunnel: [w1053] -> w1039
              tunnel: [w1052] -> w1038
              frame #0 {
                n543 = Wait (ms)(milliseconds to wait=u32 1000) -> ()  [unwired: 1 out]
              }
            }
            n544 = local read "ESP Axis"() -> (w1040:i32)
            n545 = local read "ESP_t0"() -> (w1042:dbl)
            n546 = call "Read Actual Position.vi"("error in (no error)"=w1038, "Axis (1)"=w1040, "VISA resource name"=w1039) -> ("error out"=w1033:errorcluster, "Position (units)"=w1035:dbl, "VISA resource name out"=w1037:refnum<visa-resource-name>)  [unwired: 2 in]
            n547 = call "mm2time.vi"("fs?"=TRUE, "Offset (mm)"=w1042, "distance (mm)"=w1035) -> ("time in fs/ps seconds"=w1036:dbl)
            n548 = call <vilib>:"Clear Errors.vi"("error in (no error)"=w1033) -> ("error out"=w1034:errorcluster)  [unwired: 5 in, 1 out]
            n549 = local write "ESP_pos"(w1035) -> ()
            n550 = local write "ESP_delay"(w1036) -> ()
            n551 = Send Notification(notification=TRUE, notifier=w1044, error in (no error)=w1034) -> (error out=w1045:errorcluster)  [unwired: 1 out]
          }
        }
      }
      frame "suspend" {
        n552 = Dequeue Element(queue=w1063) -> ()  [unwired: 2 in, 4 out]
      }
      frame "release" {
        n553 = Dequeue Element(queue=w1066) -> (queue out=w1064:refnum<queue>)  [unwired: 2 in, 3 out]
        n554 = call "Close.vi"("VISA resource name"=w1069) -> ("error out"=w1068:errorcluster)  [unwired: 10 in]
        n555 = Enqueue Element(queue=w1064, element="suspend") -> ()  [unwired: 2 in, 3 out]
      }
      frame "close" {
        n556 = Release Queue(queue=w1073) -> ()  [unwired: 2 in, 3 out]
      }
      frame "init" {
        n557 = Dequeue Element(queue=w1078) -> ()  [unwired: 2 in, 4 out]
        n558 = flat-sequence {
          tunnel: [w1081] -> w1075
          tunnel: [w1080] -> w1074
          tunnel: [w1085] -> w1076
          tunnel: [w1086] -> w1077
          tunnel: w1075 -> [w1086]
          tunnel: w1074 -> [w1085]
          frame #0 {
            n559 = local write "ESP_con?"(FALSE ("ESP_con?")) -> ()
          }
          frame #1 {
            n560 = call "Initialize.vi"("VISA resource name"="ESP301 VISA", "Serial Link (RS232)"=enum16{"RS232", "USB"}."RS232") -> ("VISA resource name out"=w1081:refnum<visa-resource-name>, "error out"=w1080:errorcluster)  [unwired: 7 in]
          }
          frame #2 {
            n561 = local write "ESP_con?"(TRUE ("ESP_con?")) -> ()
          }
        }
      }
    }
    "error out" <- w985
  }
  n562 = while {
    tunnel: w12 -> [w1095]
    shift-right: [w1093] -> _
    shift-left: _ -> [w1091]
    shift-right: [w1092] -> _
    shift-left: _ -> [w1090]
    shift-right: [w1088] -> _
    shift-left: 0 -> [w1089]
    tunnel: w3 -> [w1087]
    stop <- w1094 stop-if-true
    # "manip"
    n563 = Preview Queue Element(queue=w1095, timeout in ms (-1)=w1089) -> (queue out=w1098:refnum<queue>, element=w1099:string)  [unwired: 1 in, 2 out]
    n564 = Match Pattern(string=w1099, regular expression=":") -> (before substring=w1097:string, after substring=w1096:string)  [unwired: 1 in, 2 out]
    n565 = case shown="\"suspend\"" w1097 {
      tunnel: w1098 -> [_ w1111 w1138 w1185 w1223 w1229 w1238 w1243]
      tunnel: w1096 -> [_ _ w1125 w1184 _ _ _ _]
      tunnel: [_ _ _ _ _ _ TRUE _] -> w1094
      tunnel: [w1105 w1113 w1117 w1182 w1225 refnum<k5> refnum ("gateway_connection out") w1236 w1242] -> w1093
      tunnel: [w1104 w1112 w1119 w1181 w1224 w1231 w1235 w1241] -> w1092
      tunnel: w1091 -> [w1107 w1115 w1141 w1175 w1225 w1233 w1236 _]
      tunnel: w1090 -> [w1106 w1114 w1140 w1176 w1224 _ w1235 _]
      tunnel: [_ _ _ _ -1 _ _ _] -> w1088
      tunnel: w1087 -> [_ _ w1116 w1178 _ _ _ _]
      frame "idle", Default {
        n566 = call "sp_manip_get_axis_status.vi"("error in"=w1106, "gateway_connection"=w1107) -> ("error out"=w1104:errorcluster, "axis_out"=w1103:T10, "gateway_connection out"=w1105:refnum<k5>)  [unwired: 5 in, 2 out]
        n567 = for {
          tunnel: w1103 -> [w1110] mode=indexing
          tunnel: [w1109] -> w1102 mode=indexing
          tunnel: [w1108] -> w1101 mode=indexing
          n568 = Unbundle By Name(w1110) -> ("Axis_Position"=w1109:dbl, "moving"=w1108:bool)
        }
        "moving?" <- w1101
        n569 = local write "pos"(w1102) -> ()
      }
      frame "stop" {
        n570 = Dequeue Element(queue=w1111) -> ()  [unwired: 2 in, 4 out]
        n571 = call "sp_manip_abort.vi"("error in"=w1114, "gateway_connection"=w1115) -> ("error out"=w1112:errorcluster, "gateway_connection out"=w1113:refnum<k5>)  [unwired: 6 in, 2 out]
      }
      frame "rel" {
        n572 = Dequeue Element(queue=w1138) -> ()  [unwired: 2 in, 4 out]
        n573 = Match Pattern(string=w1125, regular expression=":") -> (before substring=w1124:string, after substring=w1123:string)  [unwired: 1 in, 2 out]
        n574 = Equal?(x=w1123, y="wait") -> (x = y?=w1121:bool)
        n575 = call "sp_manip_get_axis_status.vi"("error in"=w1140, "gateway_connection"=w1141) -> ("error out"=w1143:errorcluster, "axis_out"=w1130:T10, "gateway_connection out"=w1142:refnum<k5>)  [unwired: 5 in, 2 out]
        n576 = Scan From String(format string="%g_%g_%g_%g_%g_%g", input string=w1124) -> (output 1=w1137:dbl, output 2=w1136:dbl, output 3=w1135:dbl, output 4=w1134:dbl, output 5=w1133:dbl, output 6=w1132:dbl)  [unwired: 8 in, 3 out]
        n577 = for {
          tunnel: w1130 -> [w1170] mode=indexing
          tunnel: [w1169] -> w1128 mode=indexing
          tunnel: [w1168] -> w1129 mode=indexing
          n578 = Unbundle By Name(w1170) -> ("Axis_Name"=w1169:string, "Axis_Position"=w1168:dbl)
        }
        n579 = Build Array(w1137, w1136, w1135, w1134, w1133, w1132) -> (w1131:dbl[])
        n580 = Add(x=w1129, y=w1131) -> (x+y=w1127:dbl[])
        n581 = call "sp_manip_start_move.vi"("error in"=w1143, "target positions"=w1127, "axis names"=w1128, "gateway_connection"=w1142) -> ("error out"=w1120:errorcluster, "gateway_connection out"=w1118:refnum<k5>)  [unwired: 4 in, 2 out]
        n582 = case shown="True" w1121 {
          tunnel: w1120 -> [w1144 w1155]
          tunnel: [w1144 w1154] -> w1119
          tunnel: w1118 -> [w1145 w1156]
          tunnel: [w1145 w1148] -> w1117
          tunnel: w1116 -> [_ w1153]
          frame False {
          }
          frame True {
            n583 = while {
              tunnel: w1156 -> [w1162]
              tunnel: w1155 -> [w1161]
              tunnel: [w1160] -> w1149
              tunnel: [w1159] -> w1147
              stop <- w1163 continue-if-true
              n584 = call "sp_manip_get_axis_status.vi"("error in"=w1161, "gateway_connection"=w1162) -> ("error out"=w1159:errorcluster, "axis_out"=w1165:T10, "gateway_connection out"=w1160:refnum<k5>)  [unwired: 5 in, 2 out]
              n585 = for {
                tunnel: w1165 -> [w1167] mode=indexing
                tunnel: [w1166] -> w1164 mode=indexing
                n586 = Unbundle By Name(w1167) -> ("moving"=w1166:bool)
              }
              n587 = Or Array Elements(Boolean array=w1164) -> (logical OR=w1163:bool)
            }
            n588 = call "sp_manip_get_axis_status.vi"("error in"=w1147, "gateway_connection"=w1149) -> ("error out"=w1146:errorcluster, "axis_out"=w1151:T10, "gateway_connection out"=w1148:refnum<k5>)  [unwired: 5 in, 2 out]
            n589 = for {
              tunnel: w1151 -> [w1158] mode=indexing
              tunnel: [w1157] -> w1150 mode=indexing
              n590 = Unbundle By Name(w1158) -> ("Axis_Position"=w1157:dbl)
            }
            n591 = Send Notification(notification=TRUE, notifier=w1153, error in (no error)=w1146) -> (error out=w1154:errorcluster)  [unwired: 1 out]
            n592 = local write "dest"(w1150) -> ()
          }
        }
      }
      frame "abs" {
        n593 = Dequeue Element(queue=w1185) -> ()  [unwired: 2 in, 4 out]
        n594 = call "sp_manip_get_axis_status.vi"("error in"=w1176, "gateway_connection"=w1175) -> ("error out"=w1171:errorcluster, "axis_out"=w1174:T10, "gateway_connection out"=w1172:refnum<k5>)  [unwired: 5 in, 2 out]
        n595 = Match Pattern(string=w1184, regular expression=":") -> (before substring=w1188:string, after substring=w1187:string)  [unwired: 1 in, 2 out]
        n596 = Equal?(x=w1187, y="wait") -> (x = y?=w1177:bool)
        n597 = for {
          tunnel: w1174 -> [w1198] mode=indexing
          tunnel: [w1197] -> w1173 mode=indexing
          n598 = Unbundle By Name(w1198) -> ("Axis_Name"=w1197:string)
        }
        n599 = Scan From String(format string="%g_%g_%g_%g_%g_%g", input string=w1188) -> (output 1=w1194:dbl, output 2=w1193:dbl, output 3=w1192:dbl, output 4=w1191:dbl, output 5=w1190:dbl, output 6=w1189:dbl)  [unwired: 8 in, 3 out]
        n600 = Build Array(w1194, w1193, w1192, w1191, w1190, w1189) -> (w1196:dbl[])
        n601 = call "sp_manip_start_move.vi"("error in"=w1171, "target positions"=w1196, "axis names"=w1173, "gateway_connection"=w1172) -> ("error out"=w1180:errorcluster, "gateway_connection out"=w1179:refnum<k5>)  [unwired: 4 in, 2 out]
        n602 = case shown="True" w1177 {
          tunnel: w1180 -> [w1199 w1210]
          tunnel: [w1199 w1209] -> w1181
          tunnel: w1179 -> [w1200 w1211]
          tunnel: [w1200 w1202] -> w1182
          tunnel: w1178 -> [_ w1208]
          frame False {
          }
          frame True {
            n603 = while {
              tunnel: w1211 -> [w1217]
              tunnel: w1210 -> [w1216]
              tunnel: [w1215] -> w1204
              tunnel: [w1214] -> w1203
              stop <- w1218 continue-if-true
              n604 = call "sp_manip_get_axis_status.vi"("error in"=w1216, "gateway_connection"=w1217) -> ("error out"=w1214:errorcluster, "axis_out"=w1220:T10, "gateway_connection out"=w1215:refnum<k5>)  [unwired: 5 in, 2 out]
              n605 = for {
                tunnel: w1220 -> [w1222] mode=indexing
                tunnel: [w1221] -> w1219 mode=indexing
                n606 = Unbundle By Name(w1222) -> ("moving"=w1221:bool)
              }
              n607 = Or Array Elements(Boolean array=w1219) -> (logical OR=w1218:bool)
            }
            n608 = call "sp_manip_get_axis_status.vi"("error in"=w1203, "gateway_connection"=w1204) -> ("error out"=w1201:errorcluster, "axis_out"=w1206:T10, "gateway_connection out"=w1202:refnum<k5>)  [unwired: 5 in, 2 out]
            n609 = for {
              tunnel: w1206 -> [w1213] mode=indexing
              tunnel: [w1212] -> w1205 mode=indexing
              n610 = Unbundle By Name(w1213) -> ("Axis_Position"=w1212:dbl)
            }
            n611 = local write "pos"(w1205) -> ()
            n612 = Send Notification(notification=TRUE, notifier=w1208, error in (no error)=w1201) -> (error out=w1209:errorcluster)  [unwired: 1 out]
          }
        }
      }
      frame "suspend" {
        n613 = Dequeue Element(queue=w1223) -> ()  [unwired: 2 in, 4 out]
      }
      frame "release" {
        n614 = Dequeue Element(queue=w1229) -> (queue out=w1227:refnum<queue>)  [unwired: 2 in, 3 out]
        n615 = call "sp_manip_disconnect.vi"("gateway_connection"=w1233) -> ("error out"=w1232:errorcluster, "gateway_connection_out"=w1234:refnum<k5>)  [unwired: 7 in, 2 out]
        n616 = call "tcp_gateway_close_connection.vi"("error in"=w1232, "server_connection"=w1234) -> ("error out"=w1231:errorcluster)  [unwired: 5 in]
        n617 = Enqueue Element(queue=w1227, element="suspend") -> ()  [unwired: 2 in, 3 out]
      }
      frame "close" {
        n618 = Release Queue(queue=w1238) -> ()  [unwired: 2 in, 3 out]
      }
      frame "init" {
        n619 = Dequeue Element(queue=w1243) -> ()  [unwired: 2 in, 4 out]
        n620 = flat-sequence {
          tunnel: [w1246] -> w1240
          tunnel: [w1245] -> w1239
          tunnel: [w1256] -> w1241
          tunnel: [w1257] -> w1242
          tunnel: w1240 -> [w1257]
          tunnel: w1239 -> [w1256]
          frame #0 {
            n621 = local write "manip_con?"(FALSE ("manip_con?")) -> ()
          }
          frame #1 {
            n622 = call "tcp_gateway_open_connection.vi"() -> ("gateway_connection"=w1249:refnum<k5>, "error out"=w1248:errorcluster)  [unwired: 5 in, 3 out]
            n623 = call "sp_manip_connect.vi"("error in"=w1248, "gateway_connection"=w1249) -> ("error out"=w1245:errorcluster, "axis_out"=w1247:T10, "gateway_connection out"=w1246:refnum<k5>)  [unwired: 5 in, 2 out]
            n624 = for {
              tunnel: w1247 -> [w1254] mode=indexing
              tunnel: [w1253] -> w1250 mode=indexing
              tunnel: [w1252] -> w1251 mode=indexing
              n625 = Unbundle By Name(w1254) -> ("Axis_Name"=w1253:string, "Axis_Position"=w1252:dbl)
            }
            "axis" <- w1250
            "pos" <- w1251
            n626 = local write "dest"(w1251) -> ()
          }
          frame #2 {
            n627 = local write "manip_con?"(TRUE ("manip_con?")) -> ()
          }
        }
      }
    }
    "error out 2" <- w1092
  }
  n628 = while {
    tunnel: w11 -> [w1269]
    shift-right: [w1258] -> _
    shift-left: 0 -> [w1267]
    shift-right: [w1266] -> _
    shift-left: _ -> [w1265]
    shift-right: [w1264] -> _
    shift-left: _ -> [w1263]
    shift-right: [w1262] -> _
    shift-left: u32 0 ("pHandle") -> [w1261]
    tunnel: w9 -> [w1260]
    tunnel: w3 -> [w1259]
    stop <- w1268 stop-if-true
    # "phoib"
    n629 = Preview Queue Element(queue=w1269, timeout in ms (-1)=w1267) -> (queue out=w1272:refnum<queue>, element=w1273:string)  [unwired: 1 in, 2 out]
    n630 = Match Pattern(string=w1273, regular expression=":") -> (before substring=w1271:string, after substring=w1270:string)  [unwired: 1 in, 2 out]
    n631 = case shown="\"set\"" w1271 {
      tunnel: w1272 -> [_ w1330 w1385 w1402 w1420 w1434 w1439 w1444]
      tunnel: w1270 -> [_ _ w1381 _ _ _ _ _]
      tunnel: [_ _ _ _ _ TRUE _ _] -> w1268
      tunnel: [w1284 w1332 w1350 w1405 w1418 w1432 w1438 w1441] -> w1266
      tunnel: w1265 -> [w1295 w1321 w1371 w1407 w1419 w1432 w1438 _]
      tunnel: [w1283 w1331 w1366 w1404 w1417 w1430 w1436 w1440] -> w1264
      tunnel: w1263 -> [w1293 w1320 _ w1406 _ w1430 w1436 _]
      tunnel: [w1281 w1318 w1349 w1403 w1416 w1431 w1437 w1443] -> w1262
      tunnel: w1261 -> [w1281 w1318 w1369 w1403 w1415 w1431 w1437 _]
      tunnel: w1260 -> [w1282 w1311 w1347 _ _ _ _ _]
      tunnel: w1259 -> [_ _ w1365 _ _ _ _ _]
      tunnel: [_ _ _ _ _ _ -1 _] -> w1258
      frame "idle", Default {
        n632 = call "SL2_AD_DLL_Phoibos_GetDeviceState.vi"("dll_path"=w1295, "pHandle_in"=w1281, "dev_type"=DEF_dev_type."devA (analyzer)", "error in"=w1293) -> ("path out"=w1280:path, "state"=→"state":T2, "error out"=w1279:errorcluster)  [unwired: 2 in]
        n633 = for {
          tunnel: w1281 -> [w1302]
          tunnel: w1282 -> [w1300] mode=indexing
          tunnel: [w1299] -> w1292 mode=indexing
          tunnel: [w1298] -> w1284
          shift-right: [w1297] -> w1283
          shift-left: w1279 -> [w1301]
          tunnel: w1280 -> [w1296]
          n634 = call "SL2_AD_DLL_Phoibos_GetVoltage.vi"("error in"=w1301, "voltage_name"=w1300, "pHandle"=w1302, "dll path in"=w1296) -> ("error out"=w1297:errorcluster, "value"=w1299:dbl, "dll path out"=w1298:path)  [unwired: 3 in]
        }
        n635 = Index Array(array=w1292) -> (element #1=→"phoib_I_1":dbl, element #2=→"phoib_I_2":dbl, element #3=→"phoib_I_3":dbl, element #4=→"phoib_I_4":dbl, element #5=→"phoib_I_5":dbl, element #6=→"phoib_I_6":dbl, element #7=→"phoib_I_7":dbl, element #8=→"phoib_I_8":dbl, element #9=→"phoib_I_9":dbl, element #10=→"phoib_I_10":dbl)  [unwired: 10 in]
      }
      frame "set" {
        n636 = Dequeue Element(queue=w1330) -> ()  [unwired: 2 in, 4 out]
        n637 = Add(x=u32[] [251749632, 251749633, 251749634, 251749635, 251749636, 251749637, 251749638, 251749639, 251749640, 251749641, 251749642, 251749643, 251749644, 251749645, 251749646, 251749647, 251749648, 251749649, 251749650, 251749651, 251749652, 251749653, 251749654, 251749655, 251749656, 251749657, 251749658, 251749659, 251749660, 251749661, 251749662, 251749663, 251749664, 251749665, 251749666, 251749667, 251749668, 251749669, 251749670, 251749671, 251749672, 251749673, 251749674, 251749675, 251749676, 251749677, 251749678, 251749679, 251749680, 251749681, 251749682, 251749683, 251749684, 251749685, 251749686, 251749687, 251749688, 251749689, 251749690, 251749691, 251749692, 251749693, 251749694, 251749695, 251749696] ("modeIDs"), y=9984) -> (x+y=w1304:u32[])
        n638 = Multiply(x="ana_voltrange", y=12) -> (x*y=w1327:i32)
        n639 = Add(x="ana_mode", y=w1327) -> (x+y=w1324:i32)
        n640 = Index Array(array=w1304, index=w1324) -> (element=w1322:u32)
        n641 = Build Array("phoib_I_1s", "phoib_I_2s", "phoib_I_3s", "phoib_I_4s", "phoib_I_5s", "phoib_I_6s", "phoib_I_7s", "phoib_I_8s", "phoib_I_9s", "phoib_I_10s") -> (w1310:dbl[])
        n642 = call "SL2_AD_DLL_Phoibos_SetDeviceMode.vi"("pHandle"=w1318, "error in"=w1320, "value"=w1322, "dev_type"=DEF_dev_type."devA (analyzer)", "dll path in"=w1321) -> ("error out"=w1309:errorcluster, "dll path out"=w1319:path)  [unwired: 4 in]
        n643 = for {
          tunnel: w1318 -> [w1338]
          shift-right: [w1345] -> w1332
          shift-left: w1319 -> [w1342]
          tunnel: w1311 -> [w1337] mode=indexing
          tunnel: w1310 -> [w1336] mode=indexing
          shift-right: [w1344] -> w1331
          shift-left: w1309 -> [w1340]
          n644 = call "SL2_AD_DLL_Phoibos_GetVoltageRange.vi"("error in"=w1340, "voltage_name"=w1337, "pHandle"=w1338, "dll path in"=w1342) -> ("error out"=w1339:errorcluster, "min"=w1334:dbl, "max"=w1335:dbl, "dll path out"=w1341:path)  [unwired: 2 in]
          n645 = In Range and Coerce(upper limit=w1335, x=w1336, lower limit=w1334) -> (coerced(x)=w1333:dbl)  [unwired: 1 out]
          n646 = call "SL2_AD_DLL_Phoibos_SetVoltage.vi"("commit"=TRUE, "pHandle"=w1338, "error in"=w1339, "value"=w1333, "voltageName"=w1337, "dll path in"=w1341) -> ("error out"=w1344:errorcluster, "dll path out"=w1345:path)  [unwired: 3 in]
        }
      }
      frame "setsgl" {
        n647 = Dequeue Element(queue=w1385) -> ()  [unwired: 2 in, 4 out]
        n648 = Match Pattern(string=w1381, regular expression=":") -> (before substring=w1374:string, after substring=w1383:string)  [unwired: 1 in, 2 out]
        n649 = Equal?(x=w1383, y="wait") -> ()  [unwired: 1 out]
        n650 = Match Pattern(string=w1374, regular expression=":") -> (before substring=w1348:string, after substring=w1373:string)  [unwired: 1 in, 2 out]
        n651 = Fract/Exp String To Number(string=w1373) -> (number=w1372:dbl)  [unwired: 3 in, 1 out]
        n652 = call "SL2_AD_DLL_Phoibos_GetVoltageRange.vi"("voltage_name"=w1348, "pHandle"=w1369, "dll path in"=w1371) -> ("error out"=w1378:errorcluster, "min"=w1376:dbl, "max"=w1377:dbl, "dll path out"=w1379:path)  [unwired: 3 in]
        n653 = In Range and Coerce(upper limit=w1377, x=w1372, lower limit=w1376) -> (coerced(x)=w1367:dbl)  [unwired: 1 out]
        n654 = call "SL2_AD_DLL_Phoibos_SetVoltage.vi"("commit"=TRUE, "pHandle"=w1369, "error in"=w1378, "value"=w1367, "voltageName"=w1348, "dll path in"=w1379) -> ("error out"=w1368:errorcluster, "dll path out"=w1370:path)  [unwired: 3 in]
        n655 = while {
          tunnel: w1370 -> [w1401]
          tunnel: w1369 -> [w1395]
          tunnel: w1348 -> [w1400]
          tunnel: w1368 -> [w1399]
          tunnel: w1367 -> [w1398]
          tunnel: [w1395] -> w1349
          tunnel: [w1394] -> w1351
          tunnel: [w1393] -> w1353
          stop <- w1396 stop-if-true
          n656 = call "SL2_AD_DLL_Phoibos_GetVoltage.vi"("error in"=w1399, "voltage_name"=w1400, "pHandle"=w1395, "dll path in"=w1401) -> ("error out"=w1393:errorcluster, "value"=w1397:dbl, "dll path out"=w1394:path)  [unwired: 3 in]
          n657 = Equal?(x=w1398, y=w1397) -> (x = y?=w1396:bool)
        }
        n658 = for {
          tunnel: w1349 -> [w1392]
          tunnel: [w1390] -> w1354 mode=indexing
          tunnel: [w1389] -> w1350
          shift-right: [w1388] -> w1352
          shift-left: w1353 -> [w1391]
          tunnel: w1351 -> [w1387]
          tunnel: w1347 -> [w1386] mode=indexing
          n659 = call "SL2_AD_DLL_Phoibos_GetVoltage.vi"("error in"=w1391, "voltage_name"=w1386, "pHandle"=w1392, "dll path in"=w1387) -> ("error out"=w1388:errorcluster, "value"=w1390:dbl, "dll path out"=w1389:path)  [unwired: 3 in]
        }
        n660 = Index Array(array=w1354) -> (element #1=w1355:dbl, element #2=w1356:dbl, element #3=w1357:dbl, element #4=w1358:dbl, element #5=w1359:dbl, element #6=w1363:dbl, element #7=w1360:dbl, element #8=w1361:dbl, element #9=w1362:dbl, element #10=w1346:dbl)  [unwired: 10 in]
        n661 = local write "phoib_I_1"(w1355) -> ()
        n662 = local write "phoib_I_2"(w1356) -> ()
        n663 = local write "phoib_I_3"(w1357) -> ()
        n664 = local write "phoib_I_4"(w1358) -> ()
        n665 = local write "phoib_I_5"(w1359) -> ()
        n666 = local write "phoib_I_6"(w1363) -> ()
        n667 = local write "phoib_I_7"(w1360) -> ()
        n668 = local write "phoib_I_8"(w1361) -> ()
        n669 = local write "phoib_I_9"(w1362) -> ()
        n670 = local write "phoib_I_10"(w1346) -> ()
        n671 = Send Notification(notification=TRUE, notifier=w1365, error in (no error)=w1352) -> (error out=w1366:errorcluster)  [unwired: 1 out]
      }
      frame "standby" {
        w1408 = T2 0 items=["Off"=-1, "Standby"=0, "On"=1] ("state")
        n672 = Dequeue Element(queue=w1402) -> ()  [unwired: 2 in, 4 out]
        n673 = call "SL2_AD_DLL_Phoibos_SetDeviceState.vi"("pHandle_in"=w1403, "error in"=w1406, "state"=w1408, "dev_type"=DEF_dev_type."devA (analyzer)", "dll_path"=w1407) -> ("error out"=w1404:errorcluster, "path out"=w1405:path)  [unwired: 2 in]
      }
      frame "release" {
        n674 = Dequeue Element(queue=w1420) -> (queue out=w1410:refnum<queue>)  [unwired: 2 in, 3 out]
        n675 = flat-sequence {
          tunnel: w1419 -> [w1421]
          tunnel: w1415 -> [w1422]
          tunnel: [w1425] -> w1414
          tunnel: [w1424] -> w1413
          tunnel: [u32 0] -> w1412
          tunnel: [w1427] -> w1416
          tunnel: [w1428] -> w1417
          tunnel: [w1429] -> w1418
          tunnel: w1414 -> [w1429]
          tunnel: w1413 -> [w1428]
          tunnel: w1412 -> [w1427]
          frame #0 {
            n676 = call "SL2_AD_DLL_Phoibos_Shutdown.vi"("pHandle"=w1422, "dll path in"=w1421) -> ("error out"=w1424:errorcluster, "dll path out"=w1425:path)  [unwired: 4 in]
          }
          frame #1 {
            n677 = local write "phoib_con?"(FALSE ("phoib_con?")) -> ()
          }
        }
        n678 = Enqueue Element(queue=w1410, element="suspend") -> ()  [unwired: 2 in, 3 out]
      }
      frame "close" {
        n679 = Release Queue(queue=w1434) -> ()  [unwired: 2 in, 3 out]
      }
      frame "suspend" {
        n680 = Dequeue Element(queue=w1439) -> ()  [unwired: 2 in, 4 out]
      }
      frame "init" {
        n681 = Dequeue Element(queue=w1444) -> ()  [unwired: 2 in, 4 out]
        n682 = flat-sequence {
          tunnel: [w1451] -> w1442
          tunnel: [w1447] -> w1441
          tunnel: [w1446] -> w1440
          tunnel: [w1459] -> w1443
          tunnel: w1442 -> [w1459]
          frame #0 {
            n683 = local write "phoib_con?"(FALSE ("phoib_con?")) -> ()
          }
          frame #1 {
            w1450 = DEF_dev_type."devA (analyzer)" ("dev_type")
            n684 = call "GetSL2AD_VI_dllPath.vi"() -> ("error"=w1454:errorcluster, "Path"=w1455:path)  [unwired: 9 in, 1 out]
            n685 = call "SL2_AD_DLL_List_Devices.vi"("error in"=w1454, "dev_type"=w1450, "dll path in"=w1455) -> ("error out"=w1448:errorcluster, "devices"=w1457:string[], "dll path out"=w1449:path)  [unwired: 2 in]
            n686 = Index Array(array=w1457) -> (element=w1456:string)  [unwired: 1 in]
            n687 = call "SL2_AD_DLL_Phoibos_Initialize.vi"("error in"=w1448, "analyzerId"=w1456, "dll_path"=w1449) -> ("error out"=w1452:errorcluster, "pHandle"=w1451:u32, "path out"=w1453:path)  [unwired: 2 in]
            n688 = call "SL2_AD_DLL_Phoibos_ListDeviceModes.vi"("dll path in"=w1453, "dev_type"=w1450, "pHandle"=w1451, "error in"=w1452) -> ("dll path out"=w1447:path, "error out"=w1446:errorcluster)  [unwired: 1 in, 2 out]
          }
          frame #2 {
            n689 = local write "phoib_con?"(TRUE ("phoib_con?")) -> ()
          }
        }
      }
    }
    "phoib_error" <- w1264
  }
